vi "Calibration_GUI.vi"() -> ()   [LabVIEW 2012]
uses:
  Custom Controls and Typedefs/Button_GetRefImage.ctl
  Custom Controls and Typedefs/Button_AutoCalibrate.ctl
  Custom Controls and Typedefs/Flip_alongVert_Button.ctl
  Custom Controls and Typedefs/SimulationType.ctl
  Custom Controls and Typedefs/Button_RestoreCalibration.ctl
  Custom Controls and Typedefs/Clear Calibrationctl.ctl
  Custom Controls and Typedefs/CalibrationUI_States.ctl
  Custom Controls and Typedefs/CalibrationType.ctl
  Custom Controls and Typedefs/FGV_CalibrationKeyParams_Actions.ctl
  GFG/GFG Translator Wrapper/GFGTranslator_Action.ctl
  GFG/GFG Translator Wrapper/GFGTranslator_Datatype.ctl
  GFG/GFG Translator Wrapper/GFGTranslator_errors.ctl
  <vilib>/vision/Image Controls.llb/IMAQ Image.ctl
  Custom Controls and Typedefs/Calibration paramaters to Save.ctl
  Custom Controls and Typedefs/Calibration_commonParams.ctl
  SubVIs/Global_CalibrationSimulation.vi
  <vilib>/Utility/config.llb/Read Key (Double).vi
  <vilib>/vision/NI_Vision_Development_Module.lvlib
  GFG/GFG library.lvlib
  <vilib>/Utility/config.llb/NI_LVConfig.lvlib
panel:
  in  "Calibration File I/O":T3
  in  "Auto Refresh?":bool
  in  "Galvo Uncage Path":path=path "D:/Dual Channel Test Images - SciScan/2016_09_20/20160920_11_10_37_galvo_uncage_green_800nm/20160920_11_10_37_galvo_uncage_green_800nm_XYT_ch_1.bmp"
  in  "Reso Image Path":path=path "D:/Dual Channel Test Images - SciScan/2016_09_20/20160920_10_45_54_resonant_800nm_green/20160920_10_45_54_resonant_800nm_green_XYT_ch_1.bmp"
  in  "Galvo Image Path":path=path "D:/Dual Channel Test Images - SciScan/2016_09_20/20160920_11_04_00_galvo_image_green_800nm/20160920_11_04_00_galvo_image_green_800nm_XYT_ch_1.bmp"
  in  "Simulation Type - For Demo ONLY!":T4
  in  "Source Images":T5(tab)
  out "Reference Image (From Uncaging Path)":T6(plugin-control)
  in  "Uncaging Histogram":T7={"auto scale\n      Red "=TRUE, "Min Max (Red)"={0, 2047}, "Histogram"={"Starting Value"=-2011.0, "Incremental Value"=15.722656, "Histogram"=[]}} {"Min Max (Red)" scale=-1921.0..685.0}
  in  "Imaging Path Histogram":T8={"auto scale\n      Blue "=TRUE, "Min Max (Blue)"={0, 2047}, "Histogram"={"Starting Value"=0.0, "Incremental Value"=0.0, "Histogram"=[]}} {"Min Max (Blue)" scale=-32768.0..32767.0}
  out "Imaging Path Image":T6(plugin-control)
  out "Summary":string
  in  "Grab Current Image":T9
  in  "Dial":dbl(knob) scale=-5.0..5.0
  in  "Linear Zoom":cluster{"X.Zoom":dbl, "Y.Zoom":dbl}={"X.Zoom"=1.0, "Y.Zoom"=1.0} {"Y.Zoom" min=1.0 max=5.0 scale=1.0..3.0; "X.Zoom" min=1.0 max=5.0 scale=1.0..3.0}
  in  "Sinusoidal Phase Correction\n(radians)":dbl(slide)=0.6826771653543307 min=0.0 max=1.7 scale=0.0..1.7
  in  "X-Offset (Pixels)":i32(slide) scale=-256.0..256.0
  in  "Y-Offset (Pixels)":i32(slide) scale=256.0..-256.0
  in  "Offset Correction":cluster{"Dummy":dbl}
  in  "Display":enum32{"Image Overlay", "Pixel Mapping"}(tab)
  in  "Blue":bool=TRUE
  in  "Red":bool=TRUE
  out "Red-Blue Overlay":T6(plugin-control)
  out "Relationship between initial pixels and pixels after transformation":cluster{i16[], "Y Indices OUT":i16[]}[](graph)
  in  "reset zoom_Calibration_UI":bool
  in  "Clear All calibrations":bool
  in  "Read Calibration":bool
  out "Y-Pixel Mapping":i16[](array[numeric])
  out "X-Pixel Mapping":i16[](array[numeric])
  in  "Non Linear Stretch":T10={"Phase Offset (2-35%)"=25.0, "Magnitude (0-1)"=0.0} {"Magnitude (0-1)" min=0.0 max=2.0 step=1.0; "Phase Offset (2-35%)" min=2.0 max=50.0}
  in  "Flip":T11
  in  "AutoCalibrate":T12
  # "Red (Stimulation Path)"
  # "Blue (Imaging Path)"
  # "To zoom out press and hold Shift"
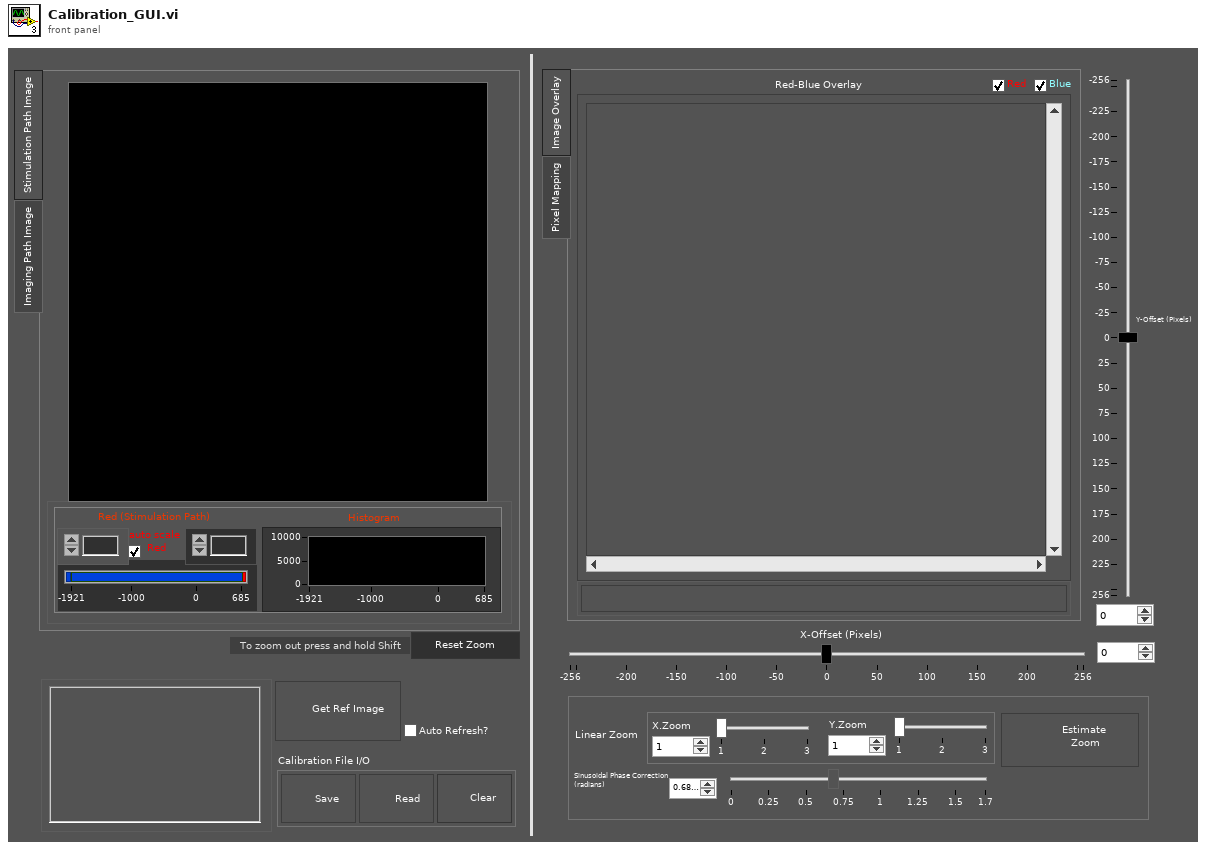
[diagram p1: front panel]
types:
  T1 = typedef "Button_RestoreCalibration.ctl" = bool
  T2 = typedef "Clear Calibrationctl.ctl" = bool
  T3 = cluster{"Save Calibration":bool, "Read Calibration":T1, "Clear Button":T2}
  T4 = typedef "SimulationType.ctl" = enum16{"None", "Uncaging Path Galvo", "Imaging Path Galvo", "Imaging Path Reso"}
  T5 = enum32{"Stimulation Path Image", "Imaging Path Image"}
  T6 = typedef "IMAQ Image.ctl" = refnum<image>
  T7 = cluster{"auto scale\n      Red ":bool, "Min Max (Red)":cluster{i16, i16}, "Histogram":cluster{"Starting Value":sgl, "Incremental Value":sgl, "Histogram":u32[]}}
  T8 = cluster{"auto scale\n      Blue ":bool, "Min Max (Blue)":cluster{i16, i16}, "Histogram":cluster{"Starting Value":sgl, "Incremental Value":sgl, "Histogram":u32[]}}
  T9 = typedef "Button_GetRefImage.ctl" = bool
  T10 = cluster{"Phase Offset (2-35%)":dbl, "Magnitude (0-1)":dbl}
  T11 = typedef "Flip_alongVert_Button.ctl" = bool
  T12 = typedef "Button_AutoCalibrate.ctl" = bool
  T13 = typedef "FGV_CalibrationKeyParams_Actions.ctl" = enum16{"Initialize", "Grab From SciScan and Store", "Read Parameters", "ReadGFGValue"}
  T14 = typedef "CalibrationType.ctl" = enum16{"None", "ImagingGalvoCalibration", "ImagingResoCalibration"}
  T15 = typedef "Image Type" = u32
  T16 = typedef "CalibrationUI_States.ctl" = enum16{"SciScan Disconnected", "Uncaging Galvo", "Imaging Galvo", "Imaging Reso", "Unknown System"}
  T17 = typedef "Calibration paramaters to Save.ctl" = cluster{"General_Parameters":cluster{"SystemType":string, "Date/Time String":string}, "Corection Parameters":cluster{"X-Offset":i32, "Y-Offset":i32, "X-Zoom":dbl, "Y-Zoom":dbl, "PhaseOffset":dbl, "Magnification":dbl, "Flip":bool}, "GFG Params(Numeric)":cluster{"GFG_Varname (Numeric)":string, "GFG_Val (Numeric)":dbl}[]}
  T18 = typedef "GFGTranslator_Datatype.ctl" = enum16{"String", "Path (String)", "Numeric", "Boolean", "Set_BoolRef (use boolean data)", "Get_Variant", "Get_2DArray (I16)", "Get_Image_2DArray (I16)", "Get_Version (String)", "Get_All GFG variables (String)"}
  T19 = typedef "GFGTranslator_Action.ctl" = enum16{"Get", "Set"}
  T20 = typedef "GFGTranslator_errors.ctl" = enum16{"Success", "SciScan Not Running", "No Get Method for Selected Datatype", "No Set Method for Selected Datatype", "Variable Not Found", "Unexpected Datatype", "Data Out of Range"}
  T21 = typedef "Calibration_commonParams.ctl" = cluster{"X.ZOOM.Compensation":dbl, "Y.ZOOM.Compensation":dbl, "Reso_Phase.Correction":dbl}
  T22 = cluster{"Starting Value":sgl, "Incremental Value":sgl, "Histogram":u32[]}
  T23 = typedef "NI_LVConfig.lvlib/Config Data RefNum.ctl" = refnum<k1>
  T24 = cluster{"X-Pixel Mapping":i16[], "Y-Pixel Mapping":i16[]}
  T25 = cluster{"Left (X) pixels dropped":i32, "Right (X) pixels dropped":i32}
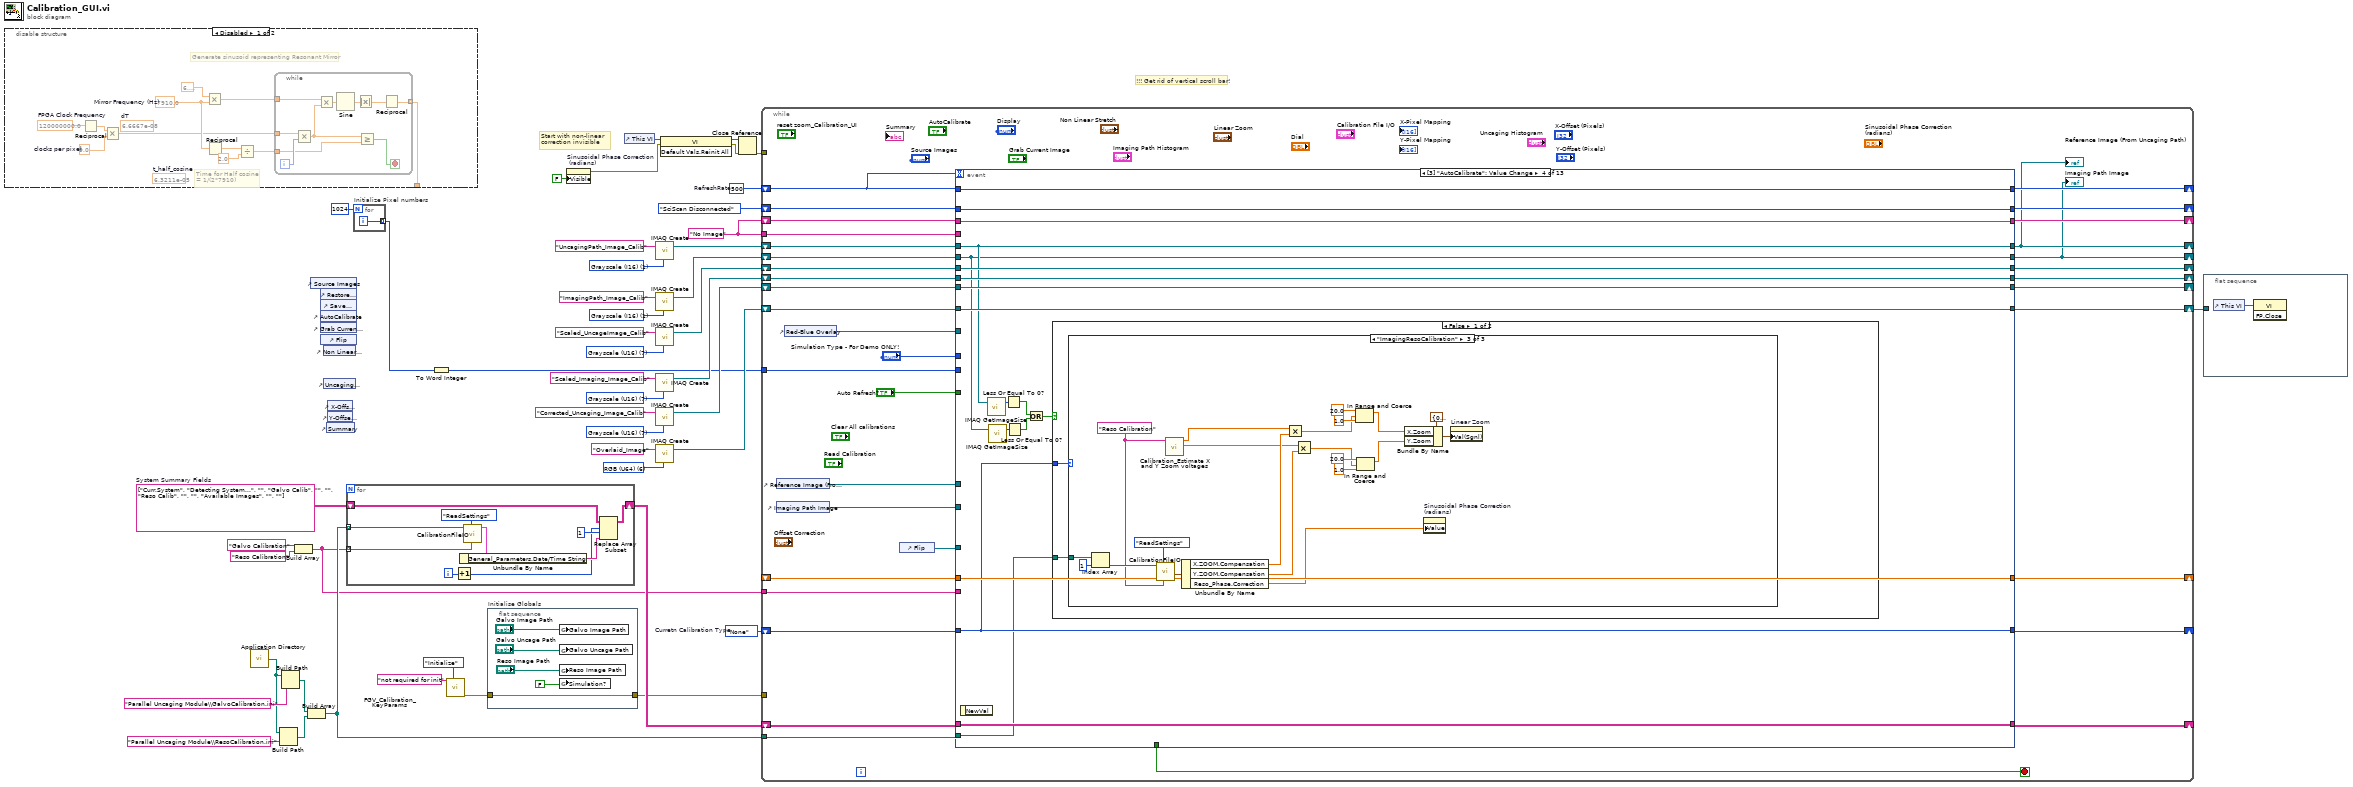
[diagram p0: block diagram]
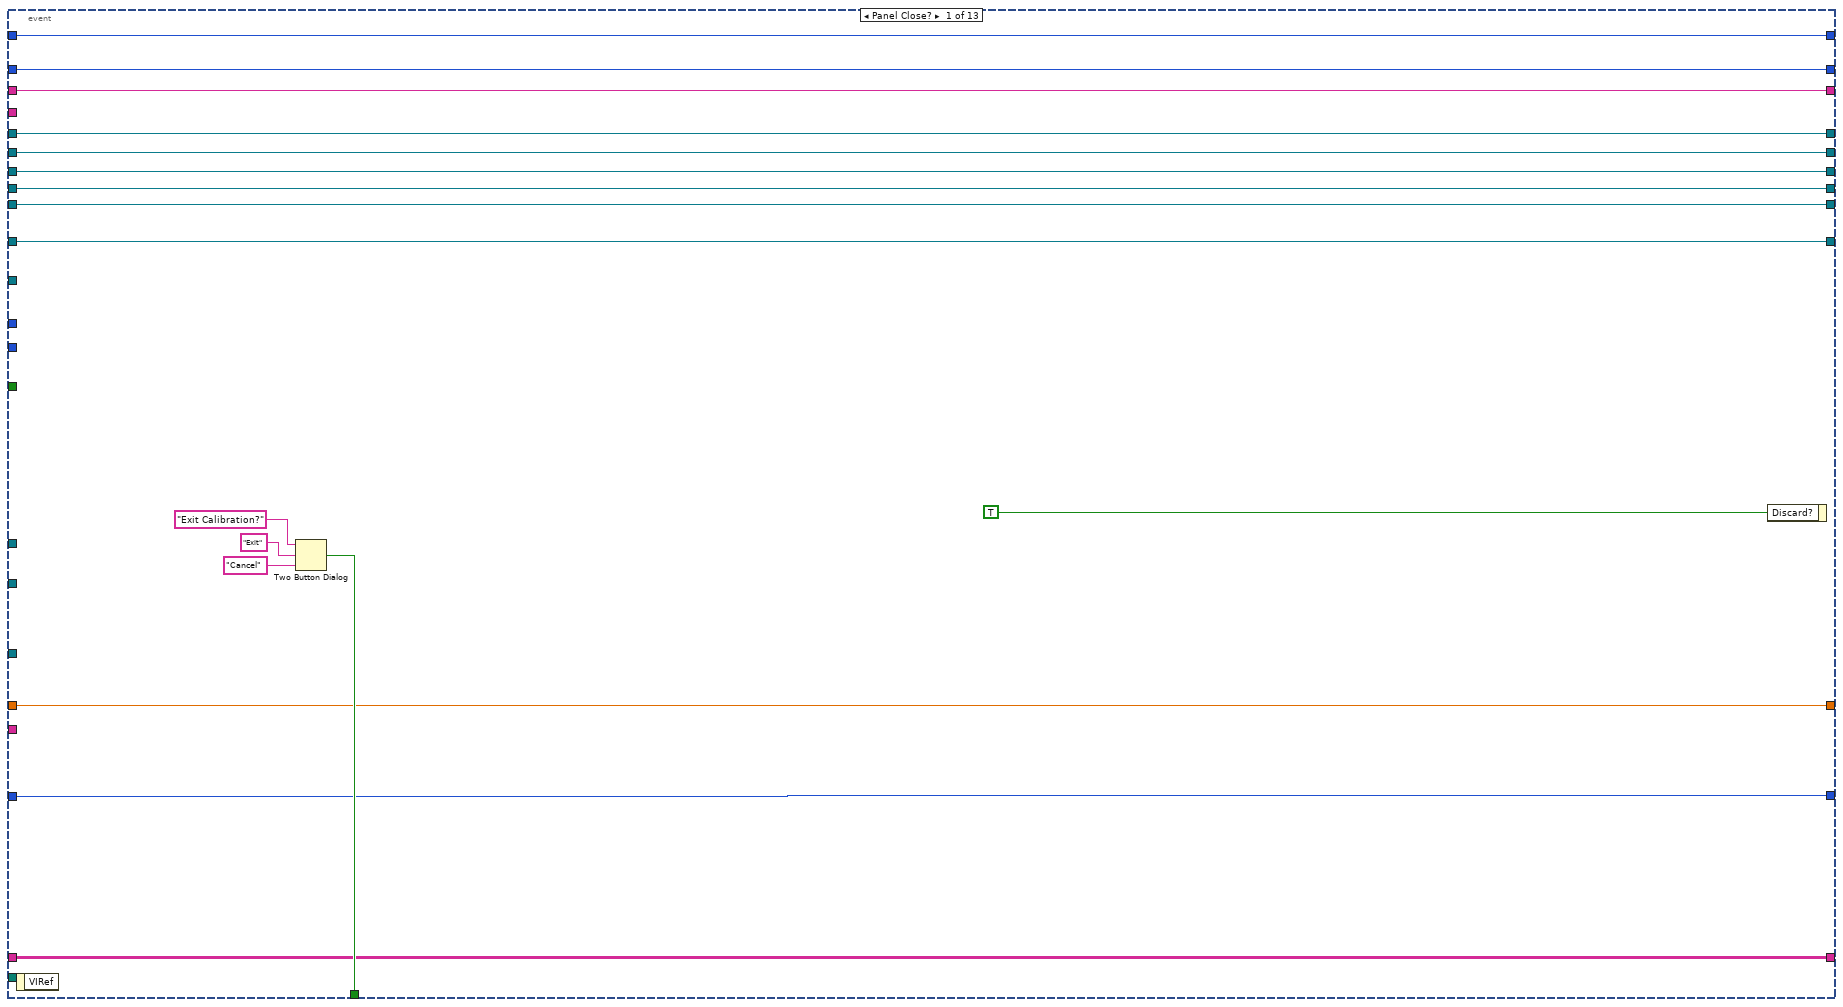
[diagram p3: hidden frame]
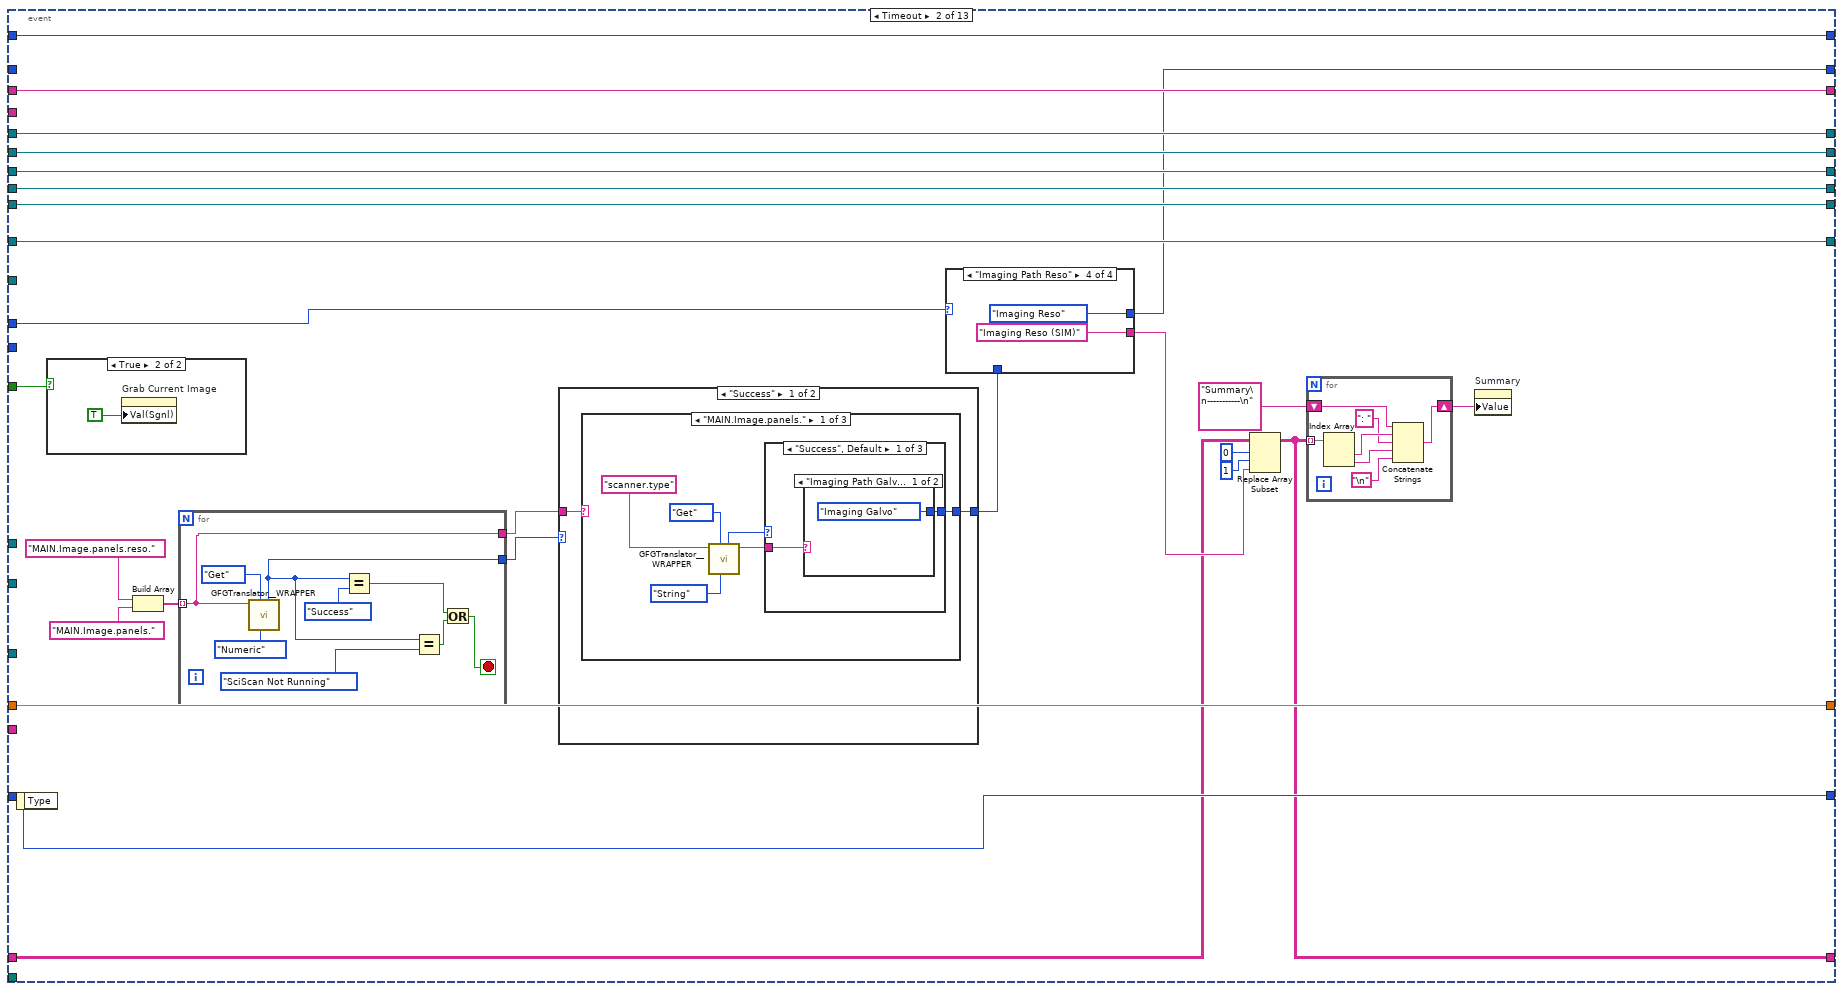
[diagram p4: hidden frame]
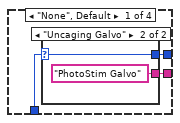
[diagram p5: hidden frame]
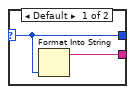
[diagram p6: hidden frame]
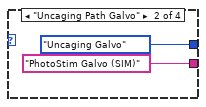
[diagram p7: hidden frame]
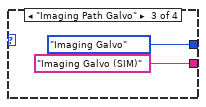
[diagram p8: hidden frame]
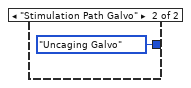
[diagram p10: hidden frame]
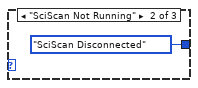
[diagram p11: hidden frame]
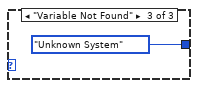
[diagram p12: hidden frame]
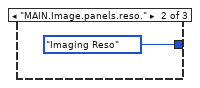
[diagram p13: hidden frame]
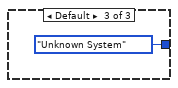
[diagram p14: hidden frame]
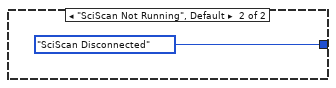
[diagram p15: hidden frame]
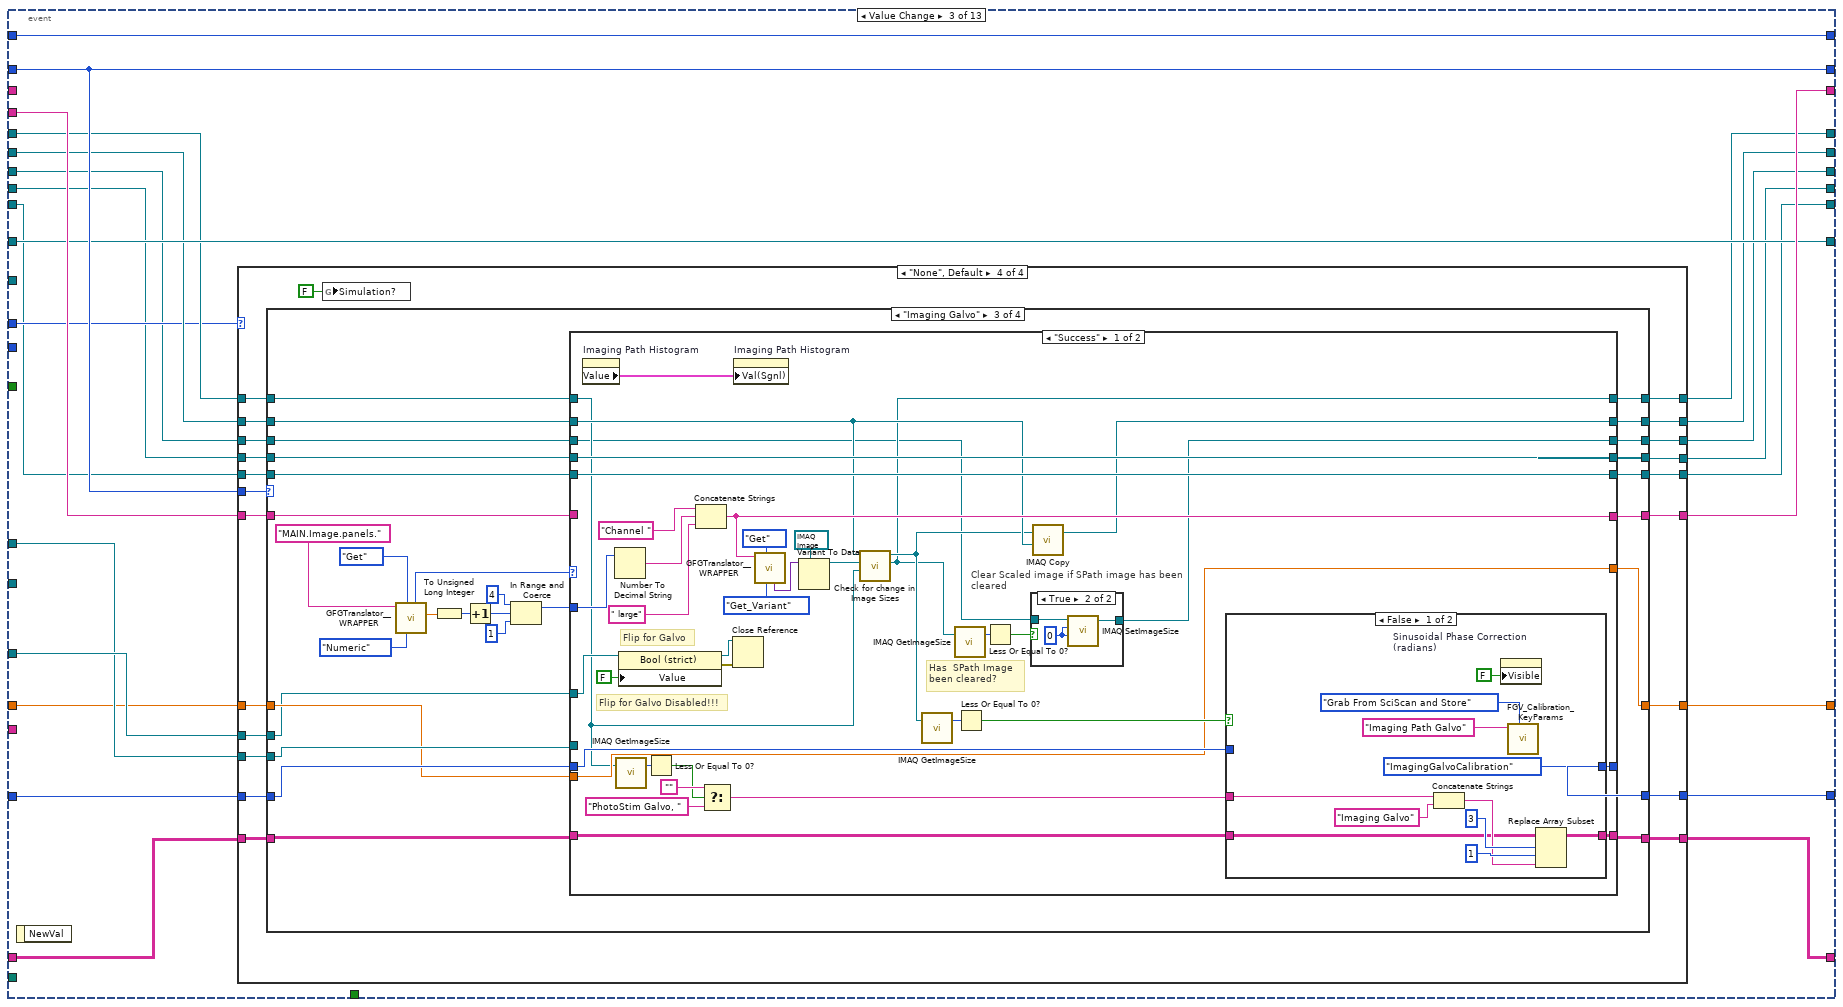
[diagram p16: hidden frame]
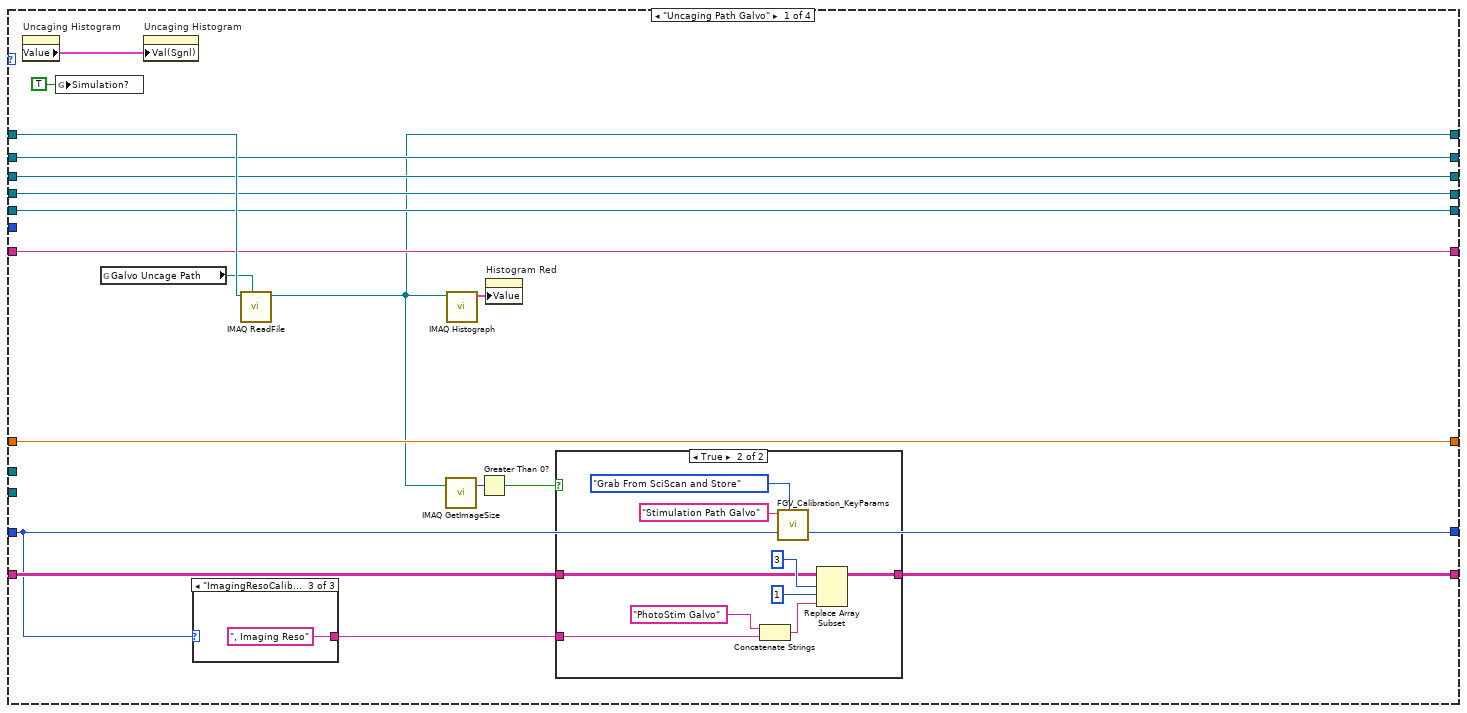
[diagram p17: hidden frame]
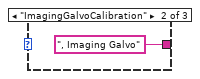
[diagram p20: hidden frame]
diagram:
  w21 = CalibrationType."None"  # Curretn Calibration Type
  w27 = T15 7 items=["Grayscale (U8)", "Grayscale (I16)", "Grayscale (SGL)", "Complex (CSG)", "RGB (U32)", "HSL (U32)", "RGB (U64)", "Grayscale (U16)"] ("Image Type")
  w30 = T15 7 items=["Grayscale (U8)", "Grayscale (I16)", "Grayscale (SGL)", "Complex (CSG)", "RGB (U32)", "HSL (U32)", "RGB (U64)", "Grayscale (U16)"] ("Image Type")
  w32 = T15 7 items=["Grayscale (U8)", "Grayscale (I16)", "Grayscale (SGL)", "Complex (CSG)", "RGB (U32)", "HSL (U32)", "RGB (U64)", "Grayscale (U16)"] ("Image Type")
  w36 = T15 1 items=["Grayscale (U8)", "Grayscale (I16)", "Grayscale (SGL)", "Complex (CSG)", "RGB (U32)", "HSL (U32)", "RGB (U64)", "Grayscale (U16)"] ("Image Type")
  w38 = T15 6 items=["Grayscale (U8)", "Grayscale (I16)", "Grayscale (SGL)", "Complex (CSG)", "RGB (U32)", "HSL (U32)", "RGB (U64)", "Grayscale (U16)"] ("Image Type")
  w39 = T15 1 items=["Grayscale (U8)", "Grayscale (I16)", "Grayscale (SGL)", "Complex (CSG)", "RGB (U32)", "HSL (U32)", "RGB (U64)", "Grayscale (U16)"] ("Image Type")
  w42 = "No Image"
  w44 = string[][] [["Curr.System", "Detecting System...", ""], ["Galvo Calib", "", ""], ["Reso Calib", "", ""], ["Available Images", "", ""]]  # System Summary Fields
  w47 = 500  # RefreshRate
  # "Start with non-linear correction invisible"
  # "!!! Get rid of vertical scroll bar!"
  n1 = disable-structure shown="Disabled" {
    disable-tunnel: [w48 _] -> _
    frame Disabled {
      w50 = 9.0  # clocks per pixel
      w52 = 120000000.0  # FPGA Clock Frequency
      w54 = 7910.0  # Mirror Frequency (Hz)
      (unwired) 6.6667e-08  # dT
      (unwired) 6.3211e-05  # t_half_cosine
      # "Generate sinusoid representing Resonant Mirror"
      # "Time for Half cosine\n= 1/(2*7910)"
      n2 = Reciprocal(x=w52) -> (1/x=w51:dbl)
      n3 = Multiply(x=w51, y=w50) -> (x*y=w49:dbl)
      n4 = Multiply(x=6.283185307179586, y=w54) -> (x*y=w57:dbl)
      n5 = Reciprocal(x=w54) -> (1/x=w55:dbl)
      n6 = Divide(x=w55, y=2.0) -> (x/y=w53:dbl)
      n7 = while {
        tunnel: w49 -> [w67]
        tunnel: w57 -> [w64]
        tunnel: w53 -> [w66]
        tunnel: [w60] -> w48 mode=indexing
        i -> [w68]
        stop <- w65 stop-if-true
        n8 = Multiply(x=w67, y=w68) -> (x*y=w63:dbl)
        n9 = Multiply(x=w64, y=w63) -> (x*y=w62:dbl)
        n10 = Sine(x=w62) -> (sin(x)=w61:dbl)
        n11 = Absolute Value(x=w61) -> (abs(x)=w59:dbl)
        n12 = Greater Or Equal?(x=w63, y=w66) -> (x >= y?=w65:bool)
        n13 = Reciprocal(x=w59) -> (1/x=w60:dbl)
      }
    }
    frame Enabled {
    }
  }
  n14 = call <vilib>:"Application Directory.vi"() -> ("Application Directory"=w23:path)
  n15 = Build Path(base path=w23, name or relative path="Parallel Uncaging Module\\ResoCalibration.ini") -> (appended path=w19:path)
  n16 = Build Path(base path=w23, name or relative path="Parallel Uncaging Module\\GalvoCalibration.ini") -> (appended path=w20:path)
  n17 = Build Array("Galvo Calibration" ("Calibration Type"), "Reso Calibration" ("Calibration Type")) -> (w6:string[])
  n18 = Build Array(w20, w19) -> (w45:path[])
  n19 = control-ref of="Source Images"() -> ()  [unwired: 1 out]
  n20 = control-ref of="Restore Calibration"() -> ()  [unwired: 1 out]
  n21 = control-ref of="Save Calibration"() -> ()  [unwired: 1 out]
  n22 = control-ref of="AutoCalibrate"() -> ()  [unwired: 1 out]
  n23 = control-ref of="Grab Current Image"() -> ()  [unwired: 1 out]
  n24 = control-ref of="Flip"() -> ()  [unwired: 1 out]
  n25 = control-ref of="Non Linear Stretch"() -> ()  [unwired: 1 out]
  n26 = control-ref of="Uncaging Histogram"() -> ()  [unwired: 1 out]
  n27 = control-ref of="Summary"() -> ()  [unwired: 1 out]
  n28 = control-ref of="X-Offset (Pixels)"() -> ()  [unwired: 1 out]
  n29 = control-ref of="Y-Offset (Pixels)"() -> ()  [unwired: 1 out]
  n30 = for {
    tunnel: w45 -> [w70] mode=indexing
    shift-right: [w72] -> w43
    shift-left: w44 -> [w76]
    tunnel: w6 -> [w69] mode=indexing
    i -> [w75]
    n31 = Increment(x=w75) -> (x+1=w71:i32)
    n32 = call "CalibrationFileIO.vi"("Calibration Type"=w69, "CalibrationFileIO_command"=enum16{"WriteSettings", "ReadSettings"}."ReadSettings", "configuration file path"=w70) -> ("Calibration paramaters_OUT"=w77:T17)  [unwired: 6 in, 2 out]
    n33 = Unbundle By Name(w77) -> ("General_Parameters.Date/Time String"=w73:string)
    n34 = Replace Array Subset(array=w76, new element=w73, index (row)=w71, index (col)=1 ("disabled index (col)")) -> (w72:string[][])
  }
  n35 = for "Initialize Pixel numbers" {
    N: 1024 -> [_]
    tunnel: [w79] -> w2 mode=indexing
    i -> [w79]
  }
  n36 = To Word Integer(number=w2) -> (16bit integer=w1:i16[])
  n37 = call "FGV_Calibration_KeyParams.vi"("Action"=FGV_CalibrationKeyParams_Actions."Initialize", "System Type"="not required for init") -> ("error out"=w12:errorcluster)  [unwired: 4 in, 5 out]
  n38 = flat-sequence "Initialise Globals" {
    tunnel: w12 -> [w80]
    tunnel: [w80] -> w11
    frame #0 {
      n39 = global write "Global_CalibrationSimulation.vi" "Galvo Image Path"("Galvo Image Path") -> ()
      n40 = global write "Global_CalibrationSimulation.vi" "Galvo Uncage Path"("Galvo Uncage Path") -> ()
      n41 = global write "Global_CalibrationSimulation.vi" "Reso Image Path"("Reso Image Path") -> ()
      n42 = global write "Global_CalibrationSimulation.vi" "Simulation?"(FALSE) -> ()
    }
  }
  n43 = property on="Sinusoidal Phase Correction\n (radians)" class="Slide (strict)"("Visible"=FALSE) -> (error out=w3:errorcluster)  [unwired: 2 in, 1 out]
  n44 = control-ref of="This VI"() -> (w16:refnum<vi>)
  n45 = call "IMAQ Create"("Image Name"="UncagingPath_Image_Calib", "Image Type"=w39) -> ("New Image"=w37:T6)  [unwired: 3 in, 1 out]
  n46 = call "IMAQ Create"("Image Name"="ImagingPath_Image_Calib", "Image Type"=w36) -> ("New Image"=w17:T6)  [unwired: 3 in, 1 out]
  n47 = call "IMAQ Create"("Image Name"="Scaled_UncageImage_Calib", "Image Type"=w32) -> ("New Image"=w31:T6)  [unwired: 3 in, 1 out]
  n48 = call "IMAQ Create"("Image Name"="Scaled_Imaging_Image_Calib", "Image Type"=w30) -> ("New Image"=w28:T6)  [unwired: 3 in, 1 out]
  n49 = call "IMAQ Create"("Image Name"="Corrected_Uncaging_Image_Calib", "Image Type"=w27) -> ("New Image"=w25:T6)  [unwired: 3 in, 1 out]
  n50 = call "IMAQ Create"("Image Name"="Overlaid_Image", "Image Type"=w38) -> ("New Image"=w34:T6)  [unwired: 3 in, 1 out]
  n51 = invoke class="VI" method="Default Vals.Reinit All"(reference=w16, error in=w3) -> (reference out=w15:refnum<vi>, error out=w14:errorcluster)  [unwired: 1 in, 1 out]
  n52 = Close Reference(reference=w15, error in (no error)=w14) -> (error out=w13:errorcluster)
  n53 = while {
    shift-right: [w118] -> _
    shift-left: w47 -> [w117]
    shift-right: [w114] -> _
    shift-left: CalibrationUI_States."SciScan Disconnected" -> [w116]
    tunnel: w45 -> [w115]
    shift-right: [w112] -> _
    shift-left: w43 -> [w113]
    shift-right: [w111] -> _
    shift-left: w42 -> [w110]
    tunnel: w42 -> [w109]
    shift-right: [w91] -> w18
    shift-left: w34 -> [w106]
    shift-right: [w89] -> _
    shift-left: w17 -> [w107]
    shift-right: [w90] -> _
    shift-left: w37 -> [w108]
    shift-right: [w100] -> _
    shift-left: w31 -> [w105]
    shift-right: [w101] -> _
    shift-left: w28 -> [w103]
    shift-right: [w99] -> _
    shift-left: w25 -> [w102]
    shift-right: [w96] -> _
    shift-left: w21 -> [w97]
    shift-right: [w93] -> _
    shift-left: _ -> [w92]
    tunnel: w13 -> [_]
    tunnel: w11 -> [_]
    tunnel: w6 -> [w88]
    tunnel: w1 -> [w86]
    stop <- w119 stop-if-true
    n54 = control-ref of="Reference Image (From Uncaging Path)"() -> (w94:refnum<vi>)
    n55 = control-ref of="Imaging Path Image"() -> (w87:refnum<vi>)
    n56 = control-ref of="Red-Blue Overlay"() -> (w85:refnum<vi>)
    n57 = control-ref of="Flip"() -> (w98:refnum<vi>)
    n58 = event shown="[3] \"AutoCalibrate\": Value Change" {
      selector: _ -> [_ _ _ _ _ _ _ _ _ _ _ _ _]
      dyn-events: _ -> [_ _ _ _ _ _ _ _ _ _ _ _ _]
      timeout: w117 -> [_ _ _ _ _ _ _ _ _ _ _ _ _]
      tunnel: [w133 _ _ _ _ _ _ _ _ _ _ _ _] -> w119
      tunnel: [w132 w162 w233 w695 w756 w785 w900 w929 w952 w1095 w1162 w1265 w1281] -> w118
      tunnel: w117 -> [w132 w162 w233 w695 w756 w785 w900 w929 w952 w1095 w1162 w1265 w1281]
      tunnel: w116 -> [w130 _ w232 w694 w755 w784 w899 w928 w951 w1094 w1146 w1264 w1280]
      tunnel: w115 -> [_ _ _ w678 _ w777 w891 _ _ _ _ _ w1269]
      tunnel: [w130 w142 w232 w694 w755 w784 w899 w928 w951 w1094 w1146 w1264 w1280] -> w114
      tunnel: w113 -> [w129 w137 w214 w693 w754 w775 w898 w927 w950 w1093 w1161 w1263 w1267]
      tunnel: [w129 w139 w213 w693 w754 w774 w898 w927 w950 w1093 w1161 w1263 w1266] -> w112
      tunnel: [w128 w154 w231 w692 w753 w783 w897 w926 w949 w1092 w1160 w1262 w1279] -> w111
      tunnel: w110 -> [w128 w154 _ w692 w753 w783 w897 w926 w949 w1092 w1160 w1262 w1279]
      tunnel: w109 -> [_ _ w230 _ _ _ _ _ _ _ _ _ _]
      tunnel: w108 -> [w127 w153 w228 w685 w752 w782 w884 w925 w946 w1089 w1159 w1261 w1278]
      tunnel: w107 -> [w126 w152 w227 w683 w751 w781 w885 w924 w948 w1067 w1158 w1260 w1277]
      tunnel: w106 -> [w125 w151 w229 w691 w750 w780 w896 w923 w942 w1091 w1151 w1259 w1276]
      tunnel: [w127 w153 w225 w685 w752 w782 w884 w925 w946 w1089 w1159 w1261 w1278] -> w90
      tunnel: [w126 w152 w226 w683 w751 w781 w885 w924 w948 w1068 w1158 w1260 w1277] -> w89
      tunnel: [w125 w151 w229 w691 w750 w780 w896 w923 w942 w1091 w1144 w1259 w1276] -> w91
      tunnel: w105 -> [w124 w150 w222 w690 w749 w772 w895 w922 w941 w1085 w1156 w1258 w1275]
      tunnel: [w124 w150 w221 w690 w749 w772 w895 w922 w939 w1085 w1156 w1258 w1275] -> w100
      tunnel: "Simulation Type - For Demo ONLY!" -> [_ w144 w224 _ _ _ _ _ _ _ _ _ _]
      tunnel: w103 -> [w123 w149 w223 w689 w748 w771 w894 w921 w943 w1077 w1149 w1257 w1274]
      tunnel: [w123 w149 w220 w689 w748 w771 w894 w921 w943 w1084 w1149 w1257 w1274] -> w101
      tunnel: w102 -> [w122 w148 w219 w688 w747 w779 w893 w920 w940 w1083 w1154 w1256 w1273]
      tunnel: [w122 w148 w218 w688 w747 w779 w893 w920 w938 w1083 w1150 w1256 w1273] -> w99
      tunnel: w98 -> [_ _ w217 _ _ w776 _ _ w934 w1079 _ w1252 _]
      tunnel: w97 -> [w121 w147 w215 w679 w746 w778 w875 w919 w933 w1063 w1145 w1251 w1272]
      tunnel: [w121 w147 w216 w679 w746 w778 w875 w919 w933 w1063 w1145 w1251 w1272] -> w96
      tunnel: "Auto Refresh?" -> [_ w146 _ _ _ _ _ _ _ _ _ _ _]
      tunnel: w94 -> [_ _ w212 _ w742 _ _ _ w931 _ _ _ _]
      tunnel: [w120 w145 w211 w687 w745 w773 w888 w918 w932 w1078 w1143 w1250 w1271] -> w93
      tunnel: w92 -> [w120 w145 w210 w687 w745 w773 w888 w918 w932 w1078 w1143 w1250 w1271]
      tunnel: w88 -> [_ _ _ _ _ w761 w887 _ _ _ _ _ _]
      tunnel: w87 -> [_ _ _ _ w743 _ _ _ _ _ _ _ _]
      tunnel: w86 -> [_ _ _ _ _ _ _ _ _ _ w1142 _ _]
      tunnel: w85 -> [_ _ _ _ w740 _ _ _ _ _ _ _ _]
      event Panel Close? {
        n59 = event-data() -> ()  [unwired: 1 in, 1 out]
        n60 = Two Button Dialog(message="Exit Calibration?", 1:"Cancel" ("F button name (\"Cancel\")"), 2:"Exit" ("T button name (\"OK\")")) -> (T button?=w133:bool)
        n61 = event-data("Discard?"=TRUE) -> ()  [unwired: 1 in, 1 out]
      }
      event Timeout {
        n62 = event-data() -> ()  [unwired: 1 in, 1 out]
        n63 = case shown="True" w146 {
          frame False {
          }
          frame True {
            n64 = property on="Grab Current Image" class="Bool"("Val(Sgnl)"=TRUE) -> ()  [unwired: 2 in, 2 out]
          }
        }
        n65 = Build Array("MAIN.Image.panels.reso." ("GFG Variable Name"), "MAIN.Image.panels." ("GFG Variable Name")) -> (w159:string[])
        n66 = for {
          tunnel: [w206] -> w158
          tunnel: w159 -> [w201] mode=indexing
          tunnel: [w201] -> w157
          stop <- w202 stop-if-true
          n67 = call "GFGTranslator__WRAPPER.vi"("GFGTranslator Datatype"=GFGTranslator_Datatype."Numeric", "GFG Translator Action"=GFGTranslator_Action."Get", "GFG Variable Name"=w201) -> ("Status Output"=w206:T20)  [unwired: 3 in, 5 out]
          n68 = Equal?(x=w206, y=GFGTranslator_errors."Success") -> (x = y?=w203:bool)
          n69 = Equal?(x=w206, y=GFGTranslator_errors."SciScan Not Running") -> (x = y?=w204:bool)
          n70 = Or(x=w203, y=w204) -> (x .or. y?=w202:bool)
        }
        n71 = case shown="\"Success\"" w158 {
          tunnel: [w184 CalibrationUI_States."SciScan Disconnected"] -> w143
          tunnel: w157 -> [w185 _]
          frame "Success" {
            n72 = case shown="\"MAIN.Image.panels.\"" w185 {
              tunnel: [w187 CalibrationUI_States."Imaging Reso" CalibrationUI_States."Unknown System"] -> w184
              frame "MAIN.Image.panels." {
                n73 = call "GFGTranslator__WRAPPER.vi"("GFGTranslator Datatype"=GFGTranslator_Datatype."String", "GFG Translator Action"=GFGTranslator_Action."Get", "GFG Variable Name"="scanner.type") -> ("String_Output"=w186:string, "Status Output"=w188:T20)  [unwired: 3 in, 4 out]
                n74 = case shown="\"Success\", Default" w188 {
                  tunnel: [w193 CalibrationUI_States."SciScan Disconnected" CalibrationUI_States."Unknown System"] -> w187
                  tunnel: w186 -> [w192 _ _]
                  frame "Success", Default {
                    n75 = case shown="\"Imaging Path Galvo\", Default" w192 {
                      tunnel: [CalibrationUI_States."Imaging Galvo" CalibrationUI_States."Uncaging Galvo"] -> w193
                      frame "Imaging Path Galvo", Default {
                      }
                      frame "Stimulation Path Galvo" {
                      }
                    }
                  }
                  frame "SciScan Not Running" {
                  }
                  frame "Variable Not Found" {
                  }
                }
              }
              frame "MAIN.Image.panels.reso." {
              }
              frame Default {
              }
            }
          }
          frame "SciScan Not Running", Default {
          }
        }
        n76 = case shown="\"Imaging Path Reso\"" w144 {
          tunnel: [w163 CalibrationUI_States."Uncaging Galvo" CalibrationUI_States."Imaging Galvo" CalibrationUI_States."Imaging Reso"] -> w142
          tunnel: w143 -> [w165 _ _ _]
          tunnel: [w164 "PhotoStim Galvo (SIM)" ("GFG Variable Name") "Imaging Galvo (SIM)" ("GFG Variable Name") "Imaging Reso (SIM)" ("GFG Variable Name")] -> w138
          frame "None", Default {
            n77 = case shown="\"Uncaging Galvo\"" w165 {
              selector: w165 -> [w167 w168]
              tunnel: [w166 "PhotoStim Galvo" ("GFG Variable Name")] -> w164
              tunnel: [w167 w168] -> w163
              frame Default {
                n78 = Format Into String(w167) -> (resulting string=w166:string)  [unwired: 3 in, 1 out]
              }
              frame "Uncaging Galvo" {
              }
            }
          }
          frame "Uncaging Path Galvo" {
          }
          frame "Imaging Path Galvo" {
          }
          frame "Imaging Path Reso" {
          }
        }
        n79 = Replace Array Subset(array=w137, new element=w138, index (row)=0, index (col)=1 ("disabled index (col)")) -> (w139:string[][])
        n80 = for {
          tunnel: w139 -> [w183] mode=indexing
          shift-right: [w177] -> w156
          shift-left: "Summary\n-----------\n" ("GFG Variable Name") -> [w178]
          n81 = Index Array(array=w183) -> (element #1=w182:string, element #2=w180:string)  [unwired: 2 in]
          n82 = Concatenate Strings(w178, w182, ": " ("string"), w180, "\n") -> (w177:string)
        }
        n83 = property on="Summary" class="Str"("Value"=w156) -> ()  [unwired: 2 in, 2 out]
      }
      event Value Change {
        n84 = event-data() -> ()  [unwired: 1 in, 1 out]
        n85 = case shown="\"None\", Default" w224 {
          tunnel: w232 -> [_ _ _ w381]
          tunnel: [w249 w285 w326 w380] -> w231
          tunnel: w230 -> [w249 w285 w326 w379]
          tunnel: w228 -> [w251 w268 w308 w378]
          tunnel: w227 -> [w250 w284 w325 w377]
          tunnel: [w250 w271 w311 w376] -> w226
          tunnel: [w236 w268 w308 w375] -> w225
          tunnel: w222 -> [w247 w282 w323 w374]
          tunnel: w223 -> [w246 w283 w324 w371]
          tunnel: [w247 w282 w323 w373] -> w221
          tunnel: [w246 w283 w324 w372] -> w220
          tunnel: w219 -> [w245 w280 w321 w369]
          tunnel: [w245 w280 w321 w370] -> w218
          tunnel: w217 -> [_ w273 w313 w368]
          tunnel: [w243 w279 w320 w367] -> w216
          tunnel: w215 -> [w243 w269 w309 w366]
          tunnel: w214 -> [w244 w278 w319 w365]
          tunnel: [w241 w277 w318 w364] -> w213
          tunnel: w212 -> [_ _ _ w363]
          tunnel: [w240 w264 w305 w362] -> w211
          tunnel: w210 -> [w240 w264 w304 w361]
          frame "Uncaging Path Galvo" {
            n86 = property on="Uncaging Histogram" class="Clust (strict)"() -> ("Value"=w239:T7)  [unwired: 2 in, 2 out]
            n87 = global write "Global_CalibrationSimulation.vi" "Simulation?"(TRUE ("Simulation?")) -> ()
            n88 = global read "Global_CalibrationSimulation.vi" "Galvo Uncage Path"() -> (w237:path)
            n89 = property on="Uncaging Histogram" class="Clust (strict)"("Val(Sgnl)"=w239) -> ()  [unwired: 2 in, 2 out]
            n90 = case shown="\"ImagingResoCalibration\"" w243 {
              tunnel: [_ ", Imaging Galvo" ("regular expression") ", Imaging Reso" ("regular expression")] -> w242
              frame "None", Default {
              }
              frame "ImagingGalvoCalibration" {
              }
              frame "ImagingResoCalibration" {
              }
            }
            n91 = call "IMAQ ReadFile"("File Path"=w237, "Image"=w251) -> ("Image Out"=w236:T6)  [unwired: 5 in, 4 out]
            n92 = call "IMAQ GetImageSize"("Image"=w236) -> ("Y Resolution"=w235:i32)  [unwired: 3 in, 2 out]
            n93 = call "IMAQ Histograph"("Image"=w236) -> ("Histogram Graph"=w248:T22)  [unwired: 7 in, 3 out]
            n94 = Greater Than 0?(x=w235) -> (x > 0?=w234:bool)
            n95 = property on="Histogram Red" class="WFGraph (strict)"("Value"=w248) -> ()  [unwired: 2 in, 2 out]
            n96 = case shown="True" w234 {
              tunnel: w244 -> [w252 w259]
              tunnel: w242 -> [_ w257]
              tunnel: [w252 w255] -> w241
              frame False {
              }
              frame True {
                n97 = Concatenate Strings("PhotoStim Galvo" ("regular expression"), w257) -> (w256:string)
                n98 = call "FGV_Calibration_KeyParams.vi"("Action"=FGV_CalibrationKeyParams_Actions."Grab From SciScan and Store", "System Type"="Stimulation Path Galvo") -> ()  [unwired: 4 in, 6 out]
                n99 = Replace Array Subset(array=w259, new element=w256, index (row)=3, index (col)=1 ("disabled index (col)")) -> (w255:string[][])
              }
            }
          }
          frame "Imaging Path Galvo" {
            # "Apply Flip for Galvo"
            n100 = property on="Imaging Path Histogram" class="Clust (strict)"() -> ("Value"=w266:T8)  [unwired: 2 in, 2 out]
            n101 = global read "Global_CalibrationSimulation.vi" "Galvo Image Path"() -> (w265:path)
            n102 = global write "Global_CalibrationSimulation.vi" "Simulation?"(TRUE ("Simulation?")) -> ()
            n103 = property class="Bool (strict)"(reference=w273, "Value"=T11 TRUE) -> (reference out=w274:refnum<vi>, error out=w275:errorcluster)  [unwired: 1 in]
            n104 = property on="Imaging Path Histogram" class="Clust (strict)"("Val(Sgnl)"=w266) -> ()  [unwired: 2 in, 2 out]
            n105 = call "IMAQ ReadFile"("File Path"=w265, "Image"=w284) -> ("Image Out"=w271:T6)  [unwired: 5 in, 4 out]
            n106 = Close Reference(reference=w274, error in (no error)=w275) -> ()  [unwired: 1 out]
            n107 = call "IMAQ GetImageSize"("Image"=w271) -> ("X Resolution"=w272:i32)  [unwired: 3 in, 2 out]
            n108 = Greater Than 0?(x=w272) -> (x > 0?=w270:bool)
            n109 = call "IMAQ Histograph"("Image"=w271) -> ("Histogram Graph"=w281:T22)  [unwired: 7 in, 3 out]
            n110 = property on="Histogram" class="WFGraph (strict)"("Value"=w281) -> ()  [unwired: 2 in, 2 out]
            n111 = case shown="True" w270 {
              tunnel: [w287 w303] -> w279
              tunnel: w278 -> [w286 w298]
              tunnel: [w286 w297] -> w277
              tunnel: w269 -> [w287 _]
              tunnel: w268 -> [_ w291]
              frame False {
              }
              frame True {
                w303 = CalibrationType."ImagingGalvoCalibration"  # Curretn Calibration Type
                n112 = property on="Sinusoidal Phase Correction\n(radians)" class="Slide (strict)"("Visible"=FALSE) -> ()  [unwired: 2 in, 2 out]
                n113 = call "IMAQ GetImageSize"("Image"=w291) -> ("X Resolution"=w293:i32)  [unwired: 3 in, 2 out]
                n114 = Greater Than 0?(x=w293) -> (x > 0?=w294:bool)
                n115 = Select(t="PhotoStim Galvo, " ("regular expression"), s=w294, f="") -> (s? t:f=w292:string)
                n116 = Concatenate Strings(w292, "Imaging Galvo" ("regular expression")) -> (w300:string)
                n117 = call "FGV_Calibration_KeyParams.vi"("Action"=FGV_CalibrationKeyParams_Actions."Grab From SciScan and Store", "System Type"="Imaging Path Galvo") -> ()  [unwired: 4 in, 6 out]
                n118 = Replace Array Subset(array=w298, new element=w300, index (row)=3, index (col)=1 ("disabled index (col)")) -> (w297:string[][])
              }
            }
          }
          frame "Imaging Path Reso" {
            # "No flip for Reso"
            n119 = global read "Global_CalibrationSimulation.vi" "Reso Image Path"() -> (w306:path)
            n120 = global write "Global_CalibrationSimulation.vi" "Simulation?"(TRUE ("Simulation?")) -> ()
            n121 = property on="Imaging Path Histogram" class="Clust (strict)"() -> ("Value"=w317:T8)  [unwired: 2 in, 2 out]
            n122 = property class="Bool (strict)"(reference=w313, "Value"=T11 FALSE) -> (reference out=w314:refnum<vi>, error out=w315:errorcluster)  [unwired: 1 in]
            n123 = call "IMAQ ReadFile"("File Path"=w306, "Image"=w325) -> ("Image Out"=w311:T6)  [unwired: 5 in, 4 out]
            n124 = Close Reference(reference=w314, error in (no error)=w315) -> ()  [unwired: 1 out]
            n125 = property on="Imaging Path Histogram" class="Clust (strict)"("Val(Sgnl)"=w317) -> ()  [unwired: 2 in, 2 out]
            n126 = call "IMAQ GetImageSize"("Image"=w311) -> ("X Resolution"=w312:i32)  [unwired: 3 in, 2 out]
            n127 = Greater Than 0?(x=w312) -> (x > 0?=w310:bool)
            n128 = case shown="True" w310 {
              tunnel: [w329 CalibrationType."ImagingResoCalibration" ("Curretn Calibration Type")] -> w320
              tunnel: w319 -> [w328 w355]
              tunnel: [w328 w354] -> w318
              tunnel: w309 -> [w329 _]
              tunnel: w308 -> [_ w347]
              tunnel: w306 -> [_ w333]
              tunnel: [w327 w332] -> w305
              tunnel: w304 -> [w327 _]
              frame False {
              }
              frame True {
                n129 = call "IMAQ GetImageSize"("Image"=w347) -> ("X Resolution"=w349:i32)  [unwired: 3 in, 2 out]
                n130 = Greater Than 0?(x=w349) -> (x > 0?=w350:bool)
                n131 = Strip Path(path=w333) -> (stripped path=w340:path, name=w342:string)
                n132 = Select(t="PhotoStim Galvo, " ("regular expression"), s=w350, f="") -> (s? t:f=w348:string)
                n133 = Match Pattern(string=w342, regular expression="_ch" ("search string")) -> (before substring=w341:string)  [unwired: 1 in, 3 out]
                n134 = Concatenate Strings(w341, ".INI" ("string")) -> (w339:string)
                n135 = Build Path(base path=w340, name or relative path=w339) -> (appended path=w338:path)
                n136 = call <vilib>:"Open Config Data.vi"("configuration file path"=w338) -> ("refnum"=w337:T23)  [unwired: 8 in, 2 out]
                n137 = Concatenate Strings(w348, "Imaging Reso" ("regular expression")) -> (w357:string)
                n138 = call "FGV_Calibration_KeyParams.vi"("Action"=FGV_CalibrationKeyParams_Actions."Grab From SciScan and Store", "System Type"="Imaging Path Reso") -> ()  [unwired: 4 in, 6 out]
                n139 = call-poly <vilib>:"Read Key.vi"("section"="_", "key"="Start.Delay", "refnum"=w337) -> ("error out"=w335:errorcluster, "value"=w332:dbl, "refnum out"=w334:T23)  [unwired: 5 in, 1 out]
                n140 = Replace Array Subset(array=w355, new element=w357, index (row)=3, index (col)=1 ("disabled index (col)")) -> (w354:string[][])
                n141 = call <vilib>:"Close Config Data.vi"("error in (no error)"=w335, "refnum"=w334) -> ()  [unwired: 8 in, 2 out]
                n142 = property on="Sinusoidal Phase Correction\n(radians)" class="Slide (strict)"("Visible"=TRUE) -> ()  [unwired: 2 in, 2 out]
              }
            }
            n143 = call "IMAQ Histograph"("Image"=w311) -> ("Histogram Graph"=w322:T22)  [unwired: 7 in, 3 out]
            n144 = property on="Histogram" class="WFGraph (strict)"("Value"=w322) -> ()  [unwired: 2 in, 2 out]
          }
          frame "None", Default {
            n145 = case shown="\"Imaging Galvo\"" w381 {
              tunnel: [w390 w420 w505 w594] -> w380
              tunnel: w379 -> [w390 w419 w504 w603]
              tunnel: w378 -> [w389 w401 w503 w600]
              tunnel: w377 -> [w388 w416 w502 w599]
              tunnel: [w388 w417 w501 w596] -> w376
              tunnel: [w389 w418 w500 w595] -> w375
              tunnel: w374 -> [w387 w415 w496 w601]
              tunnel: [w387 w414 w497 w597] -> w373
              tunnel: [w386 w413 w498 w598] -> w372
              tunnel: w371 -> [w386 w412 w499 w602]
              tunnel: [w385 w410 w494 w591] -> w370
              tunnel: w369 -> [w385 w411 w495 w592]
              tunnel: w368 -> [_ w409 w482 w580]
              tunnel: [w384 w408 w493 w590] -> w367
              tunnel: w366 -> [w384 w407 w492 w589]
              tunnel: w365 -> [w383 w406 w491 w588]
              tunnel: [w383 w405 w490 w587] -> w364
              tunnel: w363 -> [_ w404 w489 _]
              tunnel: [w382 w403 w488 w586] -> w362
              tunnel: w361 -> [w382 w402 w487 w585]
              frame "SciScan Disconnected", Default {
              }
              frame "Uncaging Galvo" {
                n146 = call "GFGTranslator__WRAPPER.vi"("GFGTranslator Datatype"=GFGTranslator_Datatype."Numeric", "GFG Translator Action"=GFGTranslator_Action."Get", "GFG Variable Name"="MAIN.Image.panels.") -> ("Numeric_Output"=w397:dbl, "Status Output"=w396:T20)  [unwired: 3 in, 4 out]
                n147 = To Unsigned Long Integer(number=w397) -> (unsigned 32bit integer=w395:u32)
                n148 = Increment(x=w395) -> (x+1=w392:u32)
                n149 = In Range and Coerce(upper limit=u32 4, x=w392, lower limit=u32 1) -> (coerced(x)=w391:u32)  [unwired: 1 out]
                n150 = case shown="\"Success\"" w396 {
                  tunnel: w391 -> [w447 _]
                  tunnel: [w453 w481] -> w420
                  tunnel: w419 -> [_ w481]
                  tunnel: w401 -> [w433 w480]
                  tunnel: [w435 w480] -> w418
                  tunnel: [w424 w479] -> w417
                  tunnel: w416 -> [w432 w479]
                  tunnel: w415 -> [w452 w478]
                  tunnel: [w452 w478] -> w414
                  tunnel: [w421 w477] -> w413
                  tunnel: w412 -> [w422 w477]
                  tunnel: w411 -> [w451 w476]
                  tunnel: [w451 w476] -> w410
                  tunnel: w409 -> [_ _]
                  tunnel: [w426 w475] -> w408
                  tunnel: w407 -> [w428 w475]
                  tunnel: w406 -> [w449 w474]
                  tunnel: [w448 w474] -> w405
                  tunnel: w404 -> [_ _]
                  tunnel: [w445 w473] -> w403
                  tunnel: w402 -> [w445 w473]
                  frame "Success" {
                    # "Has  I Path Image been cleared?"
                    # "Has Imaging Path image been cleared?"
                    n151 = property on="Uncaging Histogram" class="Clust (strict)"() -> ("Value"=w446:T7)  [unwired: 2 in, 2 out]
                    n152 = Number To Decimal String(number=w447) -> (decimal integer string=w455:string)  [unwired: 1 in]
                    n153 = Concatenate Strings("Channel " ("GFG Variable Name"), w455, " large" ("string")) -> (w453:string)
                    n154 = property on="Uncaging Histogram" class="Clust (strict)"("Val(Sgnl)"=w446) -> ()  [unwired: 2 in, 2 out]
                    n155 = call "GFGTranslator__WRAPPER.vi"("GFGTranslator Datatype"=GFGTranslator_Datatype."Get_Variant", "GFG Translator Action"=GFGTranslator_Action."Get", "GFG Variable Name"=w453) -> ("Variant_Output"=w439:variant)  [unwired: 3 in, 5 out]
                    n156 = Variant To Data(type=T6 refnum ("New Image"), Variant=w439) -> (data=w434:T6)  [unwired: 1 in, 1 out]
                    n157 = call "Check for change in Image Sizes.vi"("Other optical path [Current ImRef]"=w432, "Current Optical Path [New ImRef]"=w434, "Current Optical Path [Current ImRef]"=w433) -> ("Other Optical Path [New ImRef] OUT"=w424:T6, "Current Optical Path [New ImRef] OUT"=w431:T6)  [unwired: 7 in]
                    n158 = call "IMAQ GetImageSize"("Image"=w424) -> ("Y Resolution"=w430:i32)  [unwired: 3 in, 2 out]
                    n159 = Less Or Equal To 0?(x=w430) -> (x <= 0?=w429:bool)
                    n160 = call "IMAQ Copy"("Image Dst"=w433, "Image Src"=w431) -> ("Image Dst Out"=w435:T6)  [unwired: 4 in, 1 out]
                    n161 = Select(t=CalibrationType."None", s=w429, f=w428) -> (s? t:f=w426:T14)
                    n162 = case shown="\"None\", Default" w426 {
                      tunnel: [_ ", Imaging Galvo" ("regular expression") ", Imaging Reso" ("regular expression")] -> w450
                      frame "None", Default {
                      }
                      frame "ImagingGalvoCalibration" {
                      }
                      frame "ImagingResoCalibration" {
                      }
                    }
                    n163 = call "IMAQ GetImageSize"("Image"=w424) -> ("Y Resolution"=w425:i32)  [unwired: 3 in, 2 out]
                    n164 = call "IMAQ GetImageSize"("Image"=w431) -> ("Y Resolution"=w442:i32)  [unwired: 3 in, 2 out]
                    n165 = Less Or Equal To 0?(x=w425) -> (x <= 0?=w423:bool)
                    n166 = Less Or Equal To 0?(x=w442) -> (x <= 0?=w437:bool)
                    n167 = case "Clear Scaled image if IPath image has been cleared" shown="True" w423 {
                      tunnel: w422 -> [w457 w460]
                      tunnel: [w457 w458] -> w421
                      frame False {
                      }
                      frame True {
                        w459 = 0 ("X Resolution")
                        n168 = call "IMAQ SetImageSize"("Y Resolution"=w459, "X Resolution"=w459, "Image"=w460) -> ("Image Out"=w458:T6)  [unwired: 2 in, 1 out]
                      }
                    }
                    n169 = Select(t="", s=w437, f="PhotoStim Galvo" ("regular expression")) -> (s? t:f=w436:string)
                    n170 = case shown="False" w437 {
                      tunnel: w450 -> [w467 _]
                      tunnel: w449 -> [w466 w470]
                      tunnel: [w464 w470] -> w448
                      tunnel: w436 -> [w463 _]
                      frame False {
                        n171 = Concatenate Strings(w463, w467) -> (w465:string)
                        n172 = Replace Array Subset(array=w466, new element=w465, index (row)=3, index (col)=1 ("disabled index (col)")) -> (w464:string[][])
                        n173 = call "FGV_Calibration_KeyParams.vi"("Action"=FGV_CalibrationKeyParams_Actions."Grab From SciScan and Store", "System Type"="Stimulation Path Galvo") -> ()  [unwired: 4 in, 6 out]
                      }
                      frame True {
                        # "Empty image - do nothing!"
                      }
                    }
                  }
                  frame Default {
                  }
                }
              }
              frame "Imaging Galvo" {
                n174 = call "GFGTranslator__WRAPPER.vi"("GFGTranslator Datatype"=GFGTranslator_Datatype."Numeric", "GFG Translator Action"=GFGTranslator_Action."Get", "GFG Variable Name"="MAIN.Image.panels.") -> ("Numeric_Output"=w508:dbl, "Status Output"=w507:T20)  [unwired: 3 in, 4 out]
                n175 = To Unsigned Long Integer(number=w508) -> (unsigned 32bit integer=w506:u32)
                n176 = Increment(x=w506) -> (x+1=w486:u32)
                n177 = In Range and Coerce(upper limit=u32 4, x=w486, lower limit=u32 1) -> (coerced(x)=w483:u32)  [unwired: 1 out]
                n178 = case shown="\"Success\"" w507 {
                  tunnel: w483 -> [w541 _]
                  tunnel: [w546 w579] -> w505
                  tunnel: w504 -> [_ w579]
                  tunnel: w503 -> [w517 w577]
                  tunnel: w502 -> [w519 w578]
                  tunnel: [w522 w578] -> w501
                  tunnel: [w514 w577] -> w500
                  tunnel: w499 -> [w545 w575]
                  tunnel: [w545 w575] -> w498
                  tunnel: [w512 w576] -> w497
                  tunnel: w496 -> [w513 w576]
                  tunnel: w495 -> [w544 w574]
                  tunnel: [w544 w574] -> w494
                  tunnel: [w527 w573] -> w493
                  tunnel: w492 -> [w528 w573]
                  tunnel: w491 -> [w543 w572]
                  tunnel: [w542 w572] -> w490
                  tunnel: w489 -> [_ _]
                  tunnel: [w521 w571] -> w488
                  tunnel: w487 -> [w521 w571]
                  tunnel: w482 -> [w523 _]
                  frame "Success" {
                    # "Flip for Galvo Disabled!!!"
                    # "Has  SPath Image been cleared?"
                    # "Flip for Galvo"
                    n179 = property on="Imaging Path Histogram" class="Clust (strict)"() -> ("Value"=w540:T8)  [unwired: 2 in, 2 out]
                    n180 = Number To Decimal String(number=w541) -> (decimal integer string=w548:string)  [unwired: 1 in]
                    n181 = call "IMAQ GetImageSize"("Image"=w517) -> ("Y Resolution"=w536:i32)  [unwired: 3 in, 2 out]
                    n182 = property class="Bool (strict)"(reference=w523, "Value"=T11 FALSE) -> (reference out=w524:refnum<vi>, error out=w525:errorcluster)  [unwired: 1 in]
                    n183 = Less Or Equal To 0?(x=w536) -> (x <= 0?=w535:bool)
                    n184 = Concatenate Strings("Channel " ("GFG Variable Name"), w548, " large" ("string")) -> (w546:string)
                    n185 = Select(t="", s=w535, f="PhotoStim Galvo, " ("regular expression")) -> (s? t:f=w537:string)
                    n186 = Close Reference(reference=w524, error in (no error)=w525) -> ()  [unwired: 1 out]
                    n187 = property on="Imaging Path Histogram" class="Clust (strict)"("Val(Sgnl)"=w540) -> ()  [unwired: 2 in, 2 out]
                    n188 = call "GFGTranslator__WRAPPER.vi"("GFGTranslator Datatype"=GFGTranslator_Datatype."Get_Variant", "GFG Translator Action"=GFGTranslator_Action."Get", "GFG Variable Name"=w546) -> ("Variant_Output"=w531:variant)  [unwired: 3 in, 5 out]
                    n189 = Variant To Data(type=T6 refnum ("New Image"), Variant=w531) -> (data=w520:T6)  [unwired: 1 in, 1 out]
                    n190 = call "Check for change in Image Sizes.vi"("Other optical path [Current ImRef]"=w517, "Current Optical Path [New ImRef]"=w520, "Current Optical Path [Current ImRef]"=w519) -> ("Other Optical Path [New ImRef] OUT"=w514:T6, "Current Optical Path [New ImRef] OUT"=w518:T6)  [unwired: 7 in]
                    n191 = call "IMAQ GetImageSize"("Image"=w518) -> ("Y Resolution"=w530:i32)  [unwired: 3 in, 2 out]
                    n192 = call "IMAQ GetImageSize"("Image"=w514) -> ("Y Resolution"=w516:i32)  [unwired: 3 in, 2 out]
                    n193 = Less Or Equal To 0?(x=w530) -> (x <= 0?=w529:bool)
                    n194 = Less Or Equal To 0?(x=w516) -> (x <= 0?=w515:bool)
                    n195 = case "Clear Scaled image if SPath image has been cleared" shown="True" w515 {
                      tunnel: w513 -> [w550 w553]
                      tunnel: [w550 w551] -> w512
                      frame False {
                      }
                      frame True {
                        w552 = 0 ("X Resolution")
                        n196 = call "IMAQ SetImageSize"("Y Resolution"=w552, "X Resolution"=w552, "Image"=w553) -> ("Image Out"=w551:T6)  [unwired: 2 in, 1 out]
                      }
                    }
                    n197 = call "IMAQ Copy"("Image Dst"=w519, "Image Src"=w518) -> ("Image Dst Out"=w522:T6)  [unwired: 4 in, 1 out]
                    n198 = case shown="False" w529 {
                      tunnel: w543 -> [w561 w570]
                      tunnel: [w559 w570] -> w542
                      tunnel: w537 -> [w558 _]
                      tunnel: w528 -> [_ w566]
                      tunnel: [CalibrationType."ImagingGalvoCalibration" ("Curretn Calibration Type") w565] -> w527
                      frame False {
                        n199 = Concatenate Strings(w558, "Imaging Galvo" ("regular expression")) -> (w562:string)
                        n200 = property on="Sinusoidal Phase Correction\n(radians)" class="Slide (strict)"("Visible"=FALSE) -> ()  [unwired: 2 in, 2 out]
                        n201 = call "FGV_Calibration_KeyParams.vi"("Action"=FGV_CalibrationKeyParams_Actions."Grab From SciScan and Store", "System Type"="Imaging Path Galvo") -> ()  [unwired: 4 in, 6 out]
                        n202 = Replace Array Subset(array=w561, new element=w562, index (row)=3, index (col)=1 ("disabled index (col)")) -> (w559:string[][])
                      }
                      frame True {
                        # "clear Calibration type if Galvo image cleared"
                        # "Do nothing! - No valid image"
                        n203 = Equal?(x=CalibrationType."ImagingGalvoCalibration" ("Curretn Calibration Type"), y=w566) -> (x = y?=w568:bool)
                        n204 = Select(t=CalibrationType."None" ("Curretn Calibration Type"), s=w568, f=w566) -> (s? t:f=w565:T14)
                      }
                    }
                  }
                  frame Default {
                  }
                }
              }
              frame "Imaging Reso" {
                n205 = call "GFGTranslator__WRAPPER.vi"("GFGTranslator Datatype"=GFGTranslator_Datatype."Numeric", "GFG Translator Action"=GFGTranslator_Action."Get", "GFG Variable Name"="MAIN.Image.panels.reso.") -> ("Numeric_Output"=w605:dbl, "Status Output"=w593:T20)  [unwired: 3 in, 4 out]
                n206 = To Unsigned Long Integer(number=w605) -> (unsigned 32bit integer=w604:u32)
                n207 = Increment(x=w604) -> (x+1=w582:u32)
                n208 = In Range and Coerce(upper limit=u32 4, x=w582, lower limit=u32 1) -> (coerced(x)=w581:u32)  [unwired: 1 out]
                n209 = case shown="\"Success\"" w593 {
                  tunnel: w581 -> [w639 _]
                  tunnel: [w640 w677] -> w594
                  tunnel: w603 -> [_ w677]
                  tunnel: w600 -> [w615 w675]
                  tunnel: w599 -> [w617 w676]
                  tunnel: [w621 w676] -> w596
                  tunnel: [w612 w675] -> w595
                  tunnel: w602 -> [w609 w673]
                  tunnel: [w609 w673] -> w598
                  tunnel: [w610 w674] -> w597
                  tunnel: w601 -> [w611 w674]
                  tunnel: w592 -> [w644 w672]
                  tunnel: [w644 w672] -> w591
                  tunnel: [w626 w671] -> w590
                  tunnel: w589 -> [w627 w671]
                  tunnel: w588 -> [w643 w670]
                  tunnel: [w642 w670] -> w587
                  tunnel: [w619 w669] -> w586
                  tunnel: w585 -> [_ w669]
                  tunnel: w580 -> [w625 _]
                  frame "Success" {
                    # "Has  SPath Image been cleared?"
                    # "No flip for Reso"
                    n210 = property on="Imaging Path Histogram" class="Clust (strict)"() -> ("Value"=w641:T8)  [unwired: 2 in, 2 out]
                    n211 = Number To Decimal String(number=w639) -> (decimal integer string=w646:string)  [unwired: 1 in]
                    n212 = call "IMAQ GetImageSize"("Image"=w615) -> ("Y Resolution"=w632:i32)  [unwired: 3 in, 2 out]
                    n213 = property class="Bool (strict)"(reference=w625, "Value"=T11 FALSE) -> (reference out=w622:refnum<vi>, error out=w623:errorcluster)  [unwired: 1 in]
                    n214 = Less Or Equal To 0?(x=w632) -> (x <= 0?=w631:bool)
                    n215 = Concatenate Strings("Channel " ("GFG Variable Name"), w646, " large" ("string")) -> (w640:string)
                    n216 = Close Reference(reference=w622, error in (no error)=w623) -> ()  [unwired: 1 out]
                    n217 = call "GFGTranslator__WRAPPER.vi"("GFGTranslator Datatype"=GFGTranslator_Datatype."Get_Variant", "GFG Translator Action"=GFGTranslator_Action."Get", "GFG Variable Name"=w640) -> ("Variant_Output"=w635:variant)  [unwired: 3 in, 5 out]
                    n218 = Select(t="", s=w631, f="PhotoStim Galvo, " ("regular expression")) -> (s? t:f=w628:string)
                    n219 = property on="Imaging Path Histogram" class="Clust (strict)"("Val(Sgnl)"=w641) -> ()  [unwired: 2 in, 2 out]
                    n220 = Variant To Data(type=T6 refnum ("New Image"), Variant=w635) -> (data=w618:T6)  [unwired: 1 in, 1 out]
                    n221 = call "Check for change in Image Sizes.vi"("Other optical path [Current ImRef]"=w615, "Current Optical Path [New ImRef]"=w618, "Current Optical Path [Current ImRef]"=w617) -> ("Other Optical Path [New ImRef] OUT"=w612:T6, "Current Optical Path [New ImRef] OUT"=w616:T6)  [unwired: 7 in]
                    n222 = call "IMAQ GetImageSize"("Image"=w612) -> ("Y Resolution"=w614:i32)  [unwired: 3 in, 2 out]
                    n223 = Less Or Equal To 0?(x=w614) -> (x <= 0?=w613:bool)
                    n224 = case "Clear Scaled image if SPath image has been cleared" shown="True" w613 {
                      tunnel: w611 -> [w648 w651]
                      tunnel: [w648 w649] -> w610
                      frame False {
                      }
                      frame True {
                        w650 = 0 ("X Resolution")
                        n225 = call "IMAQ SetImageSize"("Y Resolution"=w650, "X Resolution"=w650, "Image"=w651) -> ("Image Out"=w649:T6)  [unwired: 2 in, 1 out]
                      }
                    }
                    n226 = call "IMAQ GetImageSize"("Image"=w616) -> ("Y Resolution"=w630:i32)  [unwired: 3 in, 2 out]
                    n227 = Less Or Equal To 0?(x=w630) -> (x <= 0?=w629:bool)
                    n228 = call "IMAQ Copy"("Image Dst"=w617, "Image Src"=w616) -> ("Image Dst Out"=w621:T6)  [unwired: 4 in, 1 out]
                    n229 = case shown="True" w629 {
                      tunnel: w643 -> [w658 w668]
                      tunnel: [w657 w668] -> w642
                      tunnel: w628 -> [w656 _]
                      tunnel: w627 -> [_ w664]
                      tunnel: [CalibrationType."ImagingResoCalibration" ("Curretn Calibration Type") w663] -> w626
                      frame False {
                        n230 = Concatenate Strings(w656, "Imaging Reso" ("regular expression")) -> (w660:string)
                        n231 = Replace Array Subset(array=w658, new element=w660, index (row)=3, index (col)=1 ("disabled index (col)")) -> (w657:string[][])
                        n232 = call "FGV_Calibration_KeyParams.vi"("Action"=FGV_CalibrationKeyParams_Actions."Grab From SciScan and Store", "System Type"="Imaging Path Reso") -> ()  [unwired: 4 in, 6 out]
                        n233 = property on="Sinusoidal Phase Correction\n(radians)" class="Slide (strict)"("Visible"=TRUE) -> ()  [unwired: 2 in, 2 out]
                      }
                      frame True {
                        # "clear Calibration type if Reso image cleared"
                        # "Do nothing! - No valid image"
                        # "Do nothing! - No valid image"
                        n234 = Equal?(x=CalibrationType."ImagingResoCalibration" ("Curretn Calibration Type"), y=w664) -> (x = y?=w666:bool)
                        n235 = Select(t=CalibrationType."None" ("Curretn Calibration Type"), s=w666, f=w664) -> (s? t:f=w663:T14)
                      }
                    }
                    n236 = call "GFGnumericGet.vi"("Variable Name in"="Start.Delay") -> ("Numeric"=w619:dbl)  [unwired: 8 in, 2 out]
                  }
                  frame Default {
                  }
                }
              }
            }
            n237 = global write "Global_CalibrationSimulation.vi" "Simulation?"(FALSE ("Simulation?")) -> ()
          }
        }
      }
      event Value Change {
        n238 = event-data() -> ()  [unwired: 1 in, 1 out]
        n239 = call "IMAQ GetImageSize"("Image"=w685) -> ("Y Resolution"=w686:i32)  [unwired: 3 in, 2 out]
        n240 = call "IMAQ GetImageSize"("Image"=w683) -> ("Y Resolution"=w684:i32)  [unwired: 3 in, 2 out]
        n241 = Less Or Equal To 0?(x=w686) -> (x <= 0?=w682:bool)
        n242 = Less Or Equal To 0?(x=w684) -> (x <= 0?=w681:bool)
        n243 = Or(x=w682, y=w681) -> (x .or. y?=w680:bool)
        n244 = case shown="False" w680 {
          tunnel: w679 -> [w697 _]
          tunnel: w678 -> [w696 _]
          frame False {
            n245 = case shown="\"ImagingResoCalibration\"" w697 {
              tunnel: w696 -> [_ w714 w735]
              frame Default {
              }
              frame "ImagingGalvoCalibration" {
                w708 = "Galvo Calibration" ("Calibration Type")
                n246 = Index Array(array=w714, index=0) -> (element=w712:path)
                n247 = call "CalibrationFileIO.vi"("Calibration Type"=w708, "CalibrationFileIO_command"=enum16{"WriteSettings", "ReadSettings"}."ReadSettings", "configuration file path"=w712) -> ("Common Parameters OUT"=w711:T21)  [unwired: 6 in, 2 out]
                n248 = call "Calibration_Estimate X and Y Zoom voltages.vi"("System Type"=w708) -> ("Y.ZOOM_estimated"=w706:dbl, "X.ZOOM_estimated"=w707:dbl)  [unwired: 9 in]
                n249 = Unbundle By Name(w711) -> ("X.ZOOM.Compensation"=w710:dbl, "Y.ZOOM.Compensation"=w709:dbl)
                n250 = Multiply(x=w707, y=w710) -> (x*y=w703:dbl)
                n251 = Multiply(x=w706, y=w709) -> (x*y=w699:dbl)
                n252 = In Range and Coerce(upper limit=20.0, x=w703, lower limit=1.0) -> (coerced(x)=w702:dbl)  [unwired: 1 out]
                n253 = In Range and Coerce(upper limit=20.0, x=w699, lower limit=1.0) -> (coerced(x)=w698:dbl)  [unwired: 1 out]
                n254 = Bundle By Name(cluster=cluster{"X.Zoom":dbl, "Y.Zoom":dbl} {"X.Zoom"=0.0, "Y.Zoom"=0.0} ("Value (Signaling)"), "X.Zoom"=w702, "Y.Zoom"=w698) -> (w716:cluster{"X.Zoom":dbl, "Y.Zoom":dbl})
                n255 = property on="Linear Zoom" class="Clust (strict)"("Val(Sgnl)"=w716) -> ()  [unwired: 2 in, 2 out]
              }
              frame "ImagingResoCalibration" {
                w726 = "Reso Calibration" ("Calibration Type")
                n256 = Index Array(array=w735, index=1) -> (element=w733:path)
                n257 = call "CalibrationFileIO.vi"("Calibration Type"=w726, "CalibrationFileIO_command"=enum16{"WriteSettings", "ReadSettings"}."ReadSettings", "configuration file path"=w733) -> ("Common Parameters OUT"=w732:T21)  [unwired: 6 in, 2 out]
                n258 = call "Calibration_Estimate X and Y Zoom voltages.vi"("System Type"=w726) -> ("Y.ZOOM_estimated"=w727:dbl, "X.ZOOM_estimated"=w728:dbl)  [unwired: 9 in]
                n259 = Unbundle By Name(w732) -> ("X.ZOOM.Compensation"=w731:dbl, "Y.ZOOM.Compensation"=w730:dbl, "Reso_Phase.Correction"=w729:dbl)
                n260 = Multiply(x=w728, y=w731) -> (x*y=w723:dbl)
                n261 = Multiply(x=w727, y=w730) -> (x*y=w719:dbl)
                n262 = In Range and Coerce(upper limit=20.0, x=w723, lower limit=1.0) -> (coerced(x)=w722:dbl)  [unwired: 1 out]
                n263 = In Range and Coerce(upper limit=20.0, x=w719, lower limit=1.0) -> (coerced(x)=w718:dbl)  [unwired: 1 out]
                n264 = Bundle By Name(cluster=cluster{"X.Zoom":dbl, "Y.Zoom":dbl} {"X.Zoom"=0.0, "Y.Zoom"=0.0} ("Value (Signaling)"), "X.Zoom"=w722, "Y.Zoom"=w718) -> (w737:cluster{"X.Zoom":dbl, "Y.Zoom":dbl})
                n265 = property on="Sinusoidal Phase Correction\n(radians)" class="Slide (strict)"("Value"=w729) -> ()  [unwired: 2 in, 2 out]
                n266 = property on="Linear Zoom" class="Clust (strict)"("Val(Sgnl)"=w737) -> ()  [unwired: 2 in, 2 out]
              }
            }
          }
          frame True {
            n267 = One Button Dialog(message="Auto-Calibration requires images from both optical paths!\nPlease acquire both the images and try again...\n") -> ()  [unwired: 1 in, 1 out]
          }
        }
      }
      event "reset zoom_Calibration_UI": Value Change {
        n268 = event-data() -> ()  [unwired: 1 in, 1 out]
        n269 = property on="Source Images" class="TabCtl (strict)"() -> ("Value"=w744:T5)  [unwired: 2 in, 2 out]
        n270 = property class="ImageControl"(reference=w740, "Zoom to Fit Mode"=TRUE) -> ()  [unwired: 1 in, 2 out]
        n271 = case shown="\"Stimulation Path Image\", Default" w744 {
          tunnel: w743 -> [_ w760]
          tunnel: w742 -> [w757 _]
          frame "Stimulation Path Image", Default {
            n272 = property class="ImageControl"(reference=w757, "Zoom to Fit Mode"=TRUE) -> ()  [unwired: 1 in, 2 out]
          }
          frame "Imaging Path Image" {
            n273 = property class="ImageControl"(reference=w760, "Zoom to Fit Mode"=TRUE) -> ()  [unwired: 1 in, 2 out]
          }
        }
      }
      event "Calibration File I/O.Save Calibration": Value Change {
        # "Check for equal size"
        n274 = event-data() -> ()  [unwired: 1 in, 1 out]
        n275 = call "IMAQ GetImageSize"("Image"=w772) -> ("Y Resolution"=w764:i32, "X Resolution"=w765:i32)  [unwired: 3 in, 1 out]
        n276 = call "IMAQ GetImageSize"("Image"=w771) -> ("Y Resolution"=w769:i32, "X Resolution"=w770:i32)  [unwired: 3 in, 1 out]
        n277 = Greater Than 0?(x=w765) -> (x > 0?=w762:bool)
        n278 = Greater Than 0?(x=w764) -> (x > 0?=w763:bool)
        n279 = Equal?(x=w765, y=w770) -> (x = y?=w768:bool)
        n280 = Equal?(x=w764, y=w769) -> (x = y?=w767:bool)
        n281 = Compound Arithmetic op=AND(w762, w763, w768, w767) -> (w766:bool)
        n282 = case shown="True" w766 {
          tunnel: w778 -> [_ w794]
          tunnel: w777 -> [_ w793]
          tunnel: w776 -> [_ w792]
          tunnel: w775 -> [w787 w791]
          tunnel: [w787 w788] -> w774
          tunnel: w773 -> [_ w790]
          tunnel: w761 -> [_ w789]
          frame False {
            w786 = "Cannot Save Calibration! \nPlease try again with two equally sized images."  # GUI message when image size does not fit
            n283 = One Button Dialog(message=w786) -> ()  [unwired: 1 in, 1 out]
          }
          frame True {
            n284 = case shown="\"ImagingGalvoCalibration\"" w794 {
              tunnel: w793 -> [_ w834 w869]
              tunnel: w792 -> [_ w825 w860]
              tunnel: w791 -> [w799 w813 w850]
              tunnel: [w799 w812 w846] -> w788
              tunnel: w790 -> [_ _ _]
              tunnel: w789 -> [_ w810 w845]
              frame "None", Default {
                n285 = One Button Dialog(message="Either Galvo or Reso image needs to be selected") -> ()  [unwired: 1 in, 1 out]
              }
              frame "ImagingGalvoCalibration" {
                w801 = 0.0  # No phase correction for Galvo!
                w809 = 0 ("index")
                n286 = property on="Linear Zoom" class="Clust (strict)"() -> ("Value"=w807:cluster{"X.Zoom":dbl, "Y.Zoom":dbl})  [unwired: 2 in, 2 out]
                n287 = Get Date/Time In Seconds() -> (seconds since 1Jan1904=w819:timestamp)
                n288 = property on="Non Linear Stretch" class="Clust (strict)"() -> ("Value"=w806:T10)  [unwired: 2 in, 2 out]
                n289 = property on="X-Offset (Pixels)" class="Slide (strict)"() -> ("Value"=w804:i32)  [unwired: 2 in, 2 out]
                n290 = property on="Y-Offset (Pixels)" class="Slide (strict)"() -> ("Value"=w805:i32)  [unwired: 2 in, 2 out]
                n291 = property on="Sinusoidal Phase Correction\n(radians)" class="Slide (strict)" props=["Value"]() -> ()  [unwired: 2 in, 3 out]
                n292 = Format Date/Time String(seconds (now)=w819) -> (date/time string=w811:string)  [unwired: 2 in]
                n293 = Index Array(array=w834, index=w809) -> (element=w832:path)
                n294 = Index Array "Calibration Type"(array=w810, index=w809) -> (element=w808:string)
                n295 = Unbundle By Name(w806) -> ("Phase Offset (2-35%)"=w827:dbl, "Magnitude (0-1)"=w826:dbl)
                n296 = property class="Bool (strict)"(reference=w825) -> ("Value"=w824:T11)  [unwired: 1 in, 2 out]
                n297 = Unbundle By Name(w807) -> ("X.Zoom"=w829:dbl, "Y.Zoom"=w828:dbl)
                n298 = Bundle By Name(cluster=T21 {"X.ZOOM.Compensation"=1.0, "Y.ZOOM.Compensation"=1.0, "Reso_Phase.Correction"=0.0} ("Common Parameters IN"), "Reso_Phase.Correction"=w801) -> (w802:T21)
                n299 = local read "X-Pixel Mapping"() -> (w822:i16[])
                n300 = local read "Y-Pixel Mapping"() -> (w821:i16[])
                n301 = Bundle By Name(cluster=T17 {"General_Parameters"={"SystemType"="", "Date/Time String"=""}, "Corection Parameters"={"X-Offset"=0, "Y-Offset"=0, "X-Zoom"=0.0, "Y-Zoom"=0.0, "PhaseOffset"=0.0, "Magnification"=0.0, "Flip"=FALSE}, "GFG Params(Numeric)"=[]} ("Calibration paramaters_IN"), "General_Parameters.SystemType"="Galvo", "General_Parameters.Date/Time String"=w811, "Corection Parameters.X-Offset"=w804, "Corection Parameters.Y-Offset"=w805, "Corection Parameters.X-Zoom"=w829, "Corection Parameters.Y-Zoom"=w828, "Corection Parameters.PhaseOffset"=w827, "Corection Parameters.Magnification"=w826, "Corection Parameters.Flip"=w824) -> (w823:T17)
                n302 = Bundle("X-Pixel Mapping"=w822, "Y-Pixel Mapping"=w821) -> (w820:T24)  [unwired: 1 in]
                n303 = call "CalibrationFileIO.vi"("Calibration Type"=w808, "CalibrationFileIO_command"=enum16{"WriteSettings", "ReadSettings"}."WriteSettings", "Pixel Mapping to Write"=w820, "Common Parameters IN"=w802, "Calibration paramaters_IN"=w823, "configuration file path"=w832) -> ("Calibration paramaters_OUT"=w816:T17)  [unwired: 3 in, 2 out]
                n304 = Replace Array Subset(array=w813, new element=w811, index (row)=1, index (col)=1 ("disabled index (col)")) -> (w812:string[][])
                n305 = Concatenate Strings("Galvo calibration has been updated!\nTimestamp: " ("General_Parameters.SystemType"), w811) -> (w817:string)
                n306 = flat-sequence {
                  tunnel: w817 -> [w835]
                  tunnel: w816 -> [_]
                  frame #0 {
                    n307 = One Button Dialog(message=w835) -> ()  [unwired: 1 in, 1 out]
                  }
                }
              }
              frame "ImagingResoCalibration" {
                w844 = 1 ("index")
                n308 = Get Date/Time In Seconds() -> (seconds since 1Jan1904=w854:timestamp)
                n309 = property on="Linear Zoom" class="Clust (strict)"() -> ("Value"=w842:cluster{"X.Zoom":dbl, "Y.Zoom":dbl})  [unwired: 2 in, 2 out]
                n310 = property on="Y-Offset (Pixels)" class="Slide (strict)"() -> ("Value"=w839:i32)  [unwired: 2 in, 2 out]
                n311 = property on="X-Offset (Pixels)" class="Slide (strict)"() -> ("Value"=w840:i32)  [unwired: 2 in, 2 out]
                n312 = property on="Sinusoidal Phase Correction\n(radians)" class="Slide (strict)"() -> ("Value"=w837:dbl)  [unwired: 2 in, 2 out]
                n313 = property on="Non Linear Stretch" class="Clust (strict)"() -> ("Value"=w841:T10)  [unwired: 2 in, 2 out]
                n314 = Format Date/Time String(seconds (now)=w854) -> (date/time string=w847:string)  [unwired: 2 in]
                n315 = Index Array(array=w869, index=w844) -> (element=w867:path)
                n316 = Index Array "Calibration Type"(array=w845, index=w844) -> (element=w843:string)
                n317 = Bundle By Name(cluster=T21 {"X.ZOOM.Compensation"=1.0, "Y.ZOOM.Compensation"=1.0, "Reso_Phase.Correction"=0.0} ("Common Parameters IN"), "Reso_Phase.Correction"=w837) -> (w836:T21)
                n318 = property class="Bool (strict)"(reference=w860) -> ("Value"=w859:T11)  [unwired: 1 in, 2 out]
                n319 = Unbundle By Name(w842) -> ("X.Zoom"=w864:dbl, "Y.Zoom"=w863:dbl)
                n320 = Unbundle By Name(w841) -> ("Phase Offset (2-35%)"=w862:dbl, "Magnitude (0-1)"=w861:dbl)
                n321 = local read "X-Pixel Mapping"() -> (w857:i16[])
                n322 = local read "Y-Pixel Mapping"() -> (w856:i16[])
                n323 = Bundle By Name(cluster=T17 {"General_Parameters"={"SystemType"="", "Date/Time String"=""}, "Corection Parameters"={"X-Offset"=0, "Y-Offset"=0, "X-Zoom"=0.0, "Y-Zoom"=0.0, "PhaseOffset"=0.0, "Magnification"=0.0, "Flip"=FALSE}, "GFG Params(Numeric)"=[]} ("Calibration paramaters_IN"), "General_Parameters.SystemType"="Reso", "General_Parameters.Date/Time String"=w847, "Corection Parameters.X-Offset"=w840, "Corection Parameters.Y-Offset"=w839, "Corection Parameters.X-Zoom"=w864, "Corection Parameters.Y-Zoom"=w863, "Corection Parameters.PhaseOffset"=w862, "Corection Parameters.Magnification"=w861, "Corection Parameters.Flip"=w859) -> (w858:T17)
                n324 = Bundle("X-Pixel Mapping"=w857, "Y-Pixel Mapping"=w856) -> (w855:T24)  [unwired: 1 in]
                n325 = call "CalibrationFileIO.vi"("Calibration Type"=w843, "CalibrationFileIO_command"=enum16{"WriteSettings", "ReadSettings"}."WriteSettings", "Pixel Mapping to Write"=w855, "Common Parameters IN"=w836, "Calibration paramaters_IN"=w858, "configuration file path"=w867) -> ("Calibration paramaters_OUT"=w851:T17)  [unwired: 3 in, 2 out]
                n326 = Replace Array Subset(array=w850, new element=w847, index (row)=2, index (col)=1 ("disabled index (col)")) -> (w846:string[][])
                n327 = Concatenate Strings("Reso calibration has been updated!\nTimestamp: " ("General_Parameters.SystemType"), w847) -> (w852:string)
                n328 = flat-sequence {
                  tunnel: w852 -> [w870]
                  tunnel: w851 -> [_]
                  frame #0 {
                    n329 = One Button Dialog(message=w870) -> ()  [unwired: 1 in, 1 out]
                  }
                }
              }
            }
            n330 = flat-sequence {
              tunnel: w788 -> [_]
              frame #0 {
                # "Flag a Calibration Change!"
                n331 = call "GFGTranslator__WRAPPER.vi"("GFGTranslator Datatype"=GFGTranslator_Datatype."Boolean", "GFG Translator Action"=GFGTranslator_Action."Set", "Boolean_Input"=TRUE, "GFG Variable Name"="Flag_CalibrationChanged") -> ()  [unwired: 2 in, 6 out]
              }
            }
          }
        }
      }
      event Value Change {
        # "choose the max pixels (for the case if one image is empty!)"
        n332 = event-data() -> ()  [unwired: 1 in, 1 out]
        n333 = case shown="\"ImagingResoCalibration\"" w875 {
          tunnel: [0 ("x-1") 1 ("x-1")] -> w874
          frame "None", Default {
          }
          frame "ImagingResoCalibration" {
          }
        }
        n334 = call "IMAQ GetImageSize"("Image"=w885) -> ("Y Resolution"=w881:i32, "X Resolution"=w883:i32)  [unwired: 3 in, 1 out]
        n335 = call "IMAQ GetImageSize"("Image"=w884) -> ("Y Resolution"=w880:i32, "X Resolution"=w882:i32)  [unwired: 3 in, 1 out]
        n336 = Max & Min(x=w881, y=w880) -> (max(x,y)=w877:i32)  [unwired: 1 out]
        n337 = Max & Min(x=w883, y=w882) -> (max(x,y)=w878:i32)  [unwired: 1 out]
        n338 = Bundle By Name(cluster=cluster{"X Pixels":i32, "Y Pixels":i32} {"X Pixels"=0, "Y Pixels"=0} ("Current Image Pixels"), "X Pixels"=w878, "Y Pixels"=w877) -> (w876:cluster{"X Pixels":i32, "Y Pixels":i32})
        n339 = Index Array(array=w891, index=w874) -> (element=w890:path)
        n340 = Index Array(array=w887, index=w874) -> (element=w886:string)
        n341 = call "CalibrationFileIO.vi"("Current Image Pixels"=w876, "Calibration Type"=w886, "CalibrationFileIO_command"=enum16{"WriteSettings", "ReadSettings"}."ReadSettings", "configuration file path"=w890) -> ("Common Parameters OUT"=w873:T21, "Param Matches during a read"=w871:i32, "Calibration paramaters_OUT"=w889:T17)  [unwired: 5 in]
        n342 = Less Or Equal To 0?(x=w871) -> (x <= 0?=w872:bool)
        n343 = case shown="False" w872 {
          tunnel: w889 -> [w910 _]
          tunnel: w873 -> [w902 _]
          frame False {
            n344 = Unbundle By Name(w902) -> ("Reso_Phase.Correction"=w901:dbl)
            n345 = Unbundle By Name(w910) -> ("Corection Parameters.X-Offset"=w909:i32, "Corection Parameters.Y-Offset"=w908:i32)
            n346 = Unbundle By Name(w910) -> ("Corection Parameters.X-Zoom"=w905:dbl, "Corection Parameters.Y-Zoom"=w906:dbl)
            n347 = Unbundle By Name(w910) -> ("Corection Parameters.PhaseOffset"=w913:dbl, "Corection Parameters.Magnification"=w912:dbl)
            n348 = Unbundle By Name(w910) -> ("Corection Parameters.Flip"=w904:bool)
            n349 = Bundle By Name(cluster=T10 {"Phase Offset (2-35%)"=5.0, "Magnitude (0-1)"=0.0} ("Non Linear Stretch"), "Phase Offset (2-35%)"=w913, "Magnitude (0-1)"=w912) -> (w911:T10)
            n350 = Bundle By Name(cluster=cluster{"X.Zoom":dbl, "Y.Zoom":dbl} {"X.Zoom"=1.0, "Y.Zoom"=1.0} ("Linear Zoom"), "X.Zoom"=w905, "Y.Zoom"=w906) -> (w903:cluster{"X.Zoom":dbl, "Y.Zoom":dbl})
            n351 = property on="Non Linear Stretch" class="Clust (strict)"("Value"=w911) -> ()  [unwired: 2 in, 2 out]
            n352 = property on="X-Offset (Pixels)" class="Slide (strict)"("Value"=w909) -> ()  [unwired: 2 in, 2 out]
            n353 = property on="Y-Offset (Pixels)" class="Slide (strict)"("Value"=w908) -> ()  [unwired: 2 in, 2 out]
            n354 = property on="Linear Zoom" class="Clust (strict)"("Value"=w903) -> ()  [unwired: 2 in, 2 out]
            n355 = property on="Flip" class="Bool (strict)"("Val(Sgnl)"=w904) -> ()  [unwired: 2 in, 2 out]
            n356 = property on="Sinusoidal Phase Correction\n(radians)" class="Slide (strict)"("Value"=w901) -> ()  [unwired: 2 in, 2 out]
          }
          frame True {
            n357 = One Button Dialog(message="Could not find any matching calibrations!") -> ()  [unwired: 1 in, 1 out]
          }
        }
      }
      event Value Change {
        # "Trigger an Update"
        n358 = event-data() -> ()  [unwired: 1 in, 1 out]
      }
      event "Uncaging Histogram": Value Change {
        n359 = event-data() -> ("NewVal"=w947:T7)  [unwired: 1 in]
        n360 = property class="Bool (strict)"(reference=w934) -> (reference out=w935:refnum<vi>, error out=w936:errorcluster, "Value"=w937:T11)  [unwired: 1 in]
        n361 = control-ref of="Min Max (Red)"() -> (w944:refnum<vi>)
        n362 = Unbundle By Name(w947) -> ("auto scale\n      Red"=w945:bool)
        n363 = control-ref of="Histogram"() -> (w930:refnum<vi>)
        n364 = property class="Bool (strict)"(reference=w935, error in=w936, "Val(Sgnl)"=w937) -> ()  [unwired: 2 out]
        n365 = disable-structure shown="Enabled" {
          disable-tunnel: w946 -> [w979 w999]
          disable-tunnel: w945 -> [w977 w1007]
          disable-tunnel: w944 -> [w973 w1006]
          disable-tunnel: w941 -> [w972 w1003]
          disable-tunnel: w940 -> [w971 w1002]
          disable-tunnel: [w970 w1000] -> w939
          disable-tunnel: [w969 w1001] -> w938
          disable-tunnel: w931 -> [_ w1008]
          disable-tunnel: w930 -> [_ w998]
          frame Disabled {
            w976 = u32 14 items=["Default"=10, "Most Significant Bits"=11, "Full Dynamic"=12, "Downshift"=13, "Given Range"=14, "90% Dynamic"=15, "Given Percent Range"=16] ("16-bit Display Mapping:Conversion Method")
            # "Make values positive; starting from 0"
            # "Update Scaled Image"
            n366 = call "IMAQ ImageToArray"("Image"=w979) -> ("Image Pixels (I16)"=w953:i16[][])  [unwired: 3 in, 4 out]
            n367 = Array Max & Min(array=w953) -> (min value=w956:i16)  [unwired: 3 out]
            n368 = Less Than 0?(x=w956) -> (x < 0?=w957:bool)
            n369 = case shown="True" w957 {
              tunnel: w953 -> [w980 w984]
              tunnel: w956 -> [_ w983]
              tunnel: [w980 w981] -> w955
              frame False {
              }
              frame True {
                n370 = Negate(x=w983) -> (-x=w982:i16)
                n371 = Add(x=w984, y=w982) -> (x+y=w981:i16[][])
              }
            }
            n372 = Array Max & Min(array=w955) -> (max value=w974:i16, min value=w975:i16)  [unwired: 2 out]
            n373 = case shown="True" w977 {
              tunnel: w975 -> [_ w990]
              tunnel: w974 -> [_ w989]
              tunnel: w973 -> [w988 w992]
              tunnel: [w985 w989] -> w961
              tunnel: [w986 w990] -> w960
              frame False {
                n374 = property class="Slide (strict)"(reference=w988) -> ("Value"=w987:cluster{i16, i16})  [unwired: 1 in, 2 out]
                n375 = Unbundle(w987) -> (w986:i16, w985:i16)
              }
              frame True {
                n376 = Bundle(w990, w989) -> (w991:cluster{i16, i16})  [unwired: 1 in]
                n377 = property class="Slide (strict)"(reference=w992, "Value"=w991) -> ()  [unwired: 1 in, 2 out]
              }
            }
            n378 = Absolute Value(x=w960) -> (abs(x)=w963:i16)
            n379 = Absolute Value(x=w961) -> (abs(x)=w964:i16)
            n380 = In Range and Coerce(upper limit=w961, x=w955, lower limit=w960) -> (coerced(x)=w968:i16[][])  [unwired: 1 out]
            n381 = Max & Min(x=w964, y=w963) -> (max(x,y)=w962:i16)  [unwired: 1 out]
            n382 = control-ref of="Reference Image (From Uncaging Path)"() -> (w978:refnum<vi>)
            n383 = Divide(x=w968, y=w962) -> (x/y=w967:dbl[][])
            n384 = Multiply(x=w967, y=i16 255) -> (x*y=w965:dbl[][])
            n385 = To Unsigned Byte Integer(number=w965) -> (unsigned 8bit integer=w954:u8[][])
            n386 = Array Max & Min(array=w954) -> (max value=w959:u8, min value=w958:u8)  [unwired: 2 out]
            n387 = property class="ImageControl"(reference=w978, "16-bit Display Conversion Method"=w976, "16-bit Display Maximum Value"=w959, "16-bit Display Minimum Value"=w958) -> ()  [unwired: 1 in, 2 out]
            n388 = call "IMAQ ArrayToImage"("Image Pixels (U8)"=w954, "Image"=w972) -> ("Image Out"=w970:T6)  [unwired: 8 in, 1 out]
            n389 = call "IMAQ Copy"("Image Dst"=w971, "Image Src"=w970) -> ("Image Dst Out"=w969:T6)  [unwired: 4 in, 1 out]
          }
          frame Enabled {
            w1013 = u32 14 items=["Default"=10, "Most Significant Bits"=11, "Full Dynamic"=12, "Downshift"=13, "Given Range"=14, "90% Dynamic"=15, "Given Percent Range"=16] ("16-bit Display Mapping:Conversion Method")
            # "Copy normalised image to the image for transformation ('corrected image')"
            n390 = call "IMAQ ImageToArray"("Image"=w999) -> ("Image Pixels (I16)"=w1016:i16[][])  [unwired: 3 in, 4 out]
            n391 = call "IMAQ Histograph"("Image"=w999) -> ("Histogram Graph"=w997:T22)  [unwired: 7 in, 3 out]
            n392 = case shown="False" w1007 {
              tunnel: w1016 -> [w1043 w1057]
              tunnel: [w1036 w1047] -> w1015
              tunnel: [w1037 w1048] -> w1005
              tunnel: w1006 -> [w1044 w1055]
              tunnel: [w1043 w1057] -> w1004
              tunnel: w998 -> [w1039 w1052]
              tunnel: w997 -> [w1038 w1051]
              frame False {
                n393 = property class="Slide (strict)"(reference=w1044) -> (reference out=w1042:refnum<vi>, error out=w1046:errorcluster, "Value"=w1045:cluster{i16, i16})  [unwired: 1 in]
                n394 = Close Reference(reference=w1042, error in (no error)=w1046) -> ()  [unwired: 1 out]
                n395 = Unbundle(w1045) -> (w1037:i16, w1036:i16)
                n396 = property class="WFGraph (strict)"(reference=w1039, "Value"=w1038, "XScale.Minimum"=w1037, "XScale.Maximum"=w1036) -> (reference out=w1040:refnum<vi>, error out=w1041:errorcluster)  [unwired: 1 in]
                n397 = Close Reference(reference=w1040, error in (no error)=w1041) -> ()  [unwired: 1 out]
              }
              frame True {
                n398 = Array Max & Min(array=w1057) -> (max value=w1047:i16, min value=w1048:i16)  [unwired: 2 out]
                n399 = Bundle(w1048, w1047) -> (w1054:cluster{i16, i16})  [unwired: 1 in]
                n400 = property class="WFGraph (strict)"(reference=w1052, "Value"=w1051, "XScale.Minimum"=w1048, "XScale.Maximum"=w1047) -> (reference out=w1050:refnum<vi>, error out=w1049:errorcluster)  [unwired: 1 in]
                n401 = property class="Slide (strict)"(reference=w1055, "Value"=w1054, "Scale.Minimum"=w1048, "Scale.Maximum"=w1047) -> (reference out=w1053:refnum<vi>, error out=w1056:errorcluster)  [unwired: 1 in]
                n402 = Close Reference(reference=w1053, error in (no error)=w1056) -> ()  [unwired: 1 out]
                n403 = Close Reference(reference=w1050, error in (no error)=w1049) -> ()  [unwired: 1 out]
              }
            }
            n404 = To Long Integer(number=w1015) -> (32bit integer=w995:i32)
            n405 = To Long Integer(number=w1005) -> (32bit integer=w994:i32)
            n406 = To Long Integer(number=w1004) -> (32bit integer=w993:i32[][])
            n407 = Subtract "Data range"(x=w995, y=w994) -> (x-y=w1014:i32)
            n408 = disable-structure shown="Enabled" {
              disable-tunnel: w1014 -> [w1022 w1033]
              disable-tunnel: w993 -> [w1018 w1028]
              disable-tunnel: [w1017 w1031] -> w996
              frame Disabled {
                # "Make values positive; start from 0"
                # "compress data (lossy)"
                n409 = Array Max & Min(array=w1018) -> (min value=w1024:i32)  [unwired: 3 out]
                n410 = Negate(x=w1024) -> (-x=w1023:i32)
                n411 = Add(x=w1018, y=w1023) -> (x+y=w1025:i32[][])
                n412 = Divide(x=w1025, y=w1022) -> (x/y=w1021:dbl[][])
                n413 = Multiply(x=w1021, y=255.0 ("Numeric")) -> (x*y=w1019:dbl[][])
                n414 = To Unsigned Byte Integer "Normalised to 8 bit data"(number=w1019) -> (unsigned 8bit integer=w1017:u8[][])
              }
              frame Enabled {
                n415 = Array Max & Min(array=w1028) -> (min value=w1030:i32)  [unwired: 3 out]
                n416 = Negate(x=w1030) -> (-x=w1029:i32)
                n417 = Add(x=w1028, y=w1029) -> (x+y=w1027:i32[][])
                n418 = Absolute Value(x=w1033) -> (abs(x)=w1026:i32)
                n419 = Divide(x=w1027, y=w1026) -> (x/y=w1035:dbl[][])
                n420 = Multiply(x=w1035, y=65535.0 ("Numeric")) -> (x*y=w1032:dbl[][])
                n421 = To Unsigned Word Integer(number=w1032) -> (unsigned 16bit integer=w1031:u16[][])
              }
            }
            n422 = property class="ImageControl"(reference=w1008, "16-bit Display Conversion Method"=w1013, "16-bit Display Maximum Value"=w1015) -> (reference out=w1012:refnum<vi>, error out=w1011:errorcluster)  [unwired: 1 in]
            n423 = property class="ImageControl"(reference=w1012, error in=w1011, "16-bit Display Minimum Value"=w1005) -> (reference out=w1009:refnum<vi>, error out=w1010:errorcluster)
            n424 = Close Reference(reference=w1009, error in (no error)=w1010) -> ()  [unwired: 1 out]
            n425 = call "IMAQ ArrayToImage"("Image Pixels (U16)"=w996, "Image"=w1003) -> ("Image Out"=w1000:T6)  [unwired: 8 in, 1 out]
            n426 = call "IMAQ Copy"("Image Dst"=w1002, "Image Src"=w1000) -> ("Image Dst Out"=w1001:T6)  [unwired: 4 in, 1 out]
          }
        }
      }
      event "Imaging Path Histogram": Value Change {
        w1073 = u32 14 items=["Default"=10, "Most Significant Bits"=11, "Full Dynamic"=12, "Downshift"=13, "Given Range"=14, "90% Dynamic"=15, "Given Percent Range"=16] ("16-bit Display Mapping:Conversion Method")
        n427 = event-data() -> ("NewVal"=w1090:T8)  [unwired: 1 in]
        n428 = property class="Bool (strict)"(reference=w1079) -> (reference out=w1082:refnum<vi>, error out=w1081:errorcluster, "Value"=w1080:T11)  [unwired: 1 in]
        n429 = control-ref of="Imaging Path Image"() -> (w1087:refnum<vi>)
        n430 = control-ref of="Min Max (Blue)"() -> (w1086:refnum<vi>)
        n431 = Unbundle By Name(w1090) -> ("auto scale\n      Blue"=w1088:bool)
        n432 = control-ref of="Histogram"() -> (w1066:refnum<vi>)
        n433 = property class="Bool (strict)"(reference=w1082, error in=w1081, "Val(Sgnl)"=w1080) -> ()  [unwired: 2 out]
        n434 = call "IMAQ ImageToArray"("Image"=w1067) -> ("Image Pixels (I16)"=w1061:i16[][])  [unwired: 3 in, 4 out]
        n435 = call "IMAQ Histograph"("Image"=w1067) -> ("Histogram Graph"=w1065:T22)  [unwired: 7 in, 3 out]
        n436 = case shown="False" w1088 {
          tunnel: w1061 -> [w1120 w1141]
          tunnel: [w1121 w1131] -> w1076
          tunnel: [w1122 w1132] -> w1075
          tunnel: w1086 -> [w1128 w1136]
          tunnel: [w1120 w1141] -> w1062
          tunnel: w1066 -> [w1123 w1138]
          tunnel: w1065 -> [w1124 w1137]
          frame False {
            n437 = property class="Slide (strict)"(reference=w1128) -> (reference out=w1127:refnum<vi>, error out=w1130:errorcluster, "Value"=w1129:cluster{i16, i16})  [unwired: 1 in]
            n438 = Close Reference(reference=w1127, error in (no error)=w1130) -> ()  [unwired: 1 out]
            n439 = Unbundle(w1129) -> (w1122:i16, w1121:i16)
            n440 = property class="WFGraph (strict)"(reference=w1123, "Value"=w1124, "XScale.Minimum"=w1122, "XScale.Maximum"=w1121) -> (reference out=w1126:refnum<vi>, error out=w1125:errorcluster)  [unwired: 1 in]
            n441 = Close Reference(reference=w1126, error in (no error)=w1125) -> ()  [unwired: 1 out]
          }
          frame True {
            n442 = Array Max & Min(array=w1141) -> (max value=w1131:i16, min value=w1132:i16)  [unwired: 2 out]
            n443 = Bundle(w1132, w1131) -> (w1134:cluster{i16, i16})  [unwired: 1 in]
            n444 = property class="WFGraph (strict)"(reference=w1138, "Value"=w1137, "XScale.Minimum"=w1132, "XScale.Maximum"=w1131) -> (reference out=w1140:refnum<vi>, error out=w1139:errorcluster)  [unwired: 1 in]
            n445 = property class="Slide (strict)"(reference=w1136, "Value"=w1134, "Scale.Minimum"=w1132, "Scale.Maximum"=w1131) -> (reference out=w1135:refnum<vi>, error out=w1133:errorcluster)  [unwired: 1 in]
            n446 = Close Reference(reference=w1135, error in (no error)=w1133) -> ()  [unwired: 1 out]
            n447 = Close Reference(reference=w1140, error in (no error)=w1139) -> ()  [unwired: 1 out]
          }
        }
        n448 = To Long Integer(number=w1075) -> (32bit integer=w1059:i32)
        n449 = To Long Integer(number=w1076) -> (32bit integer=w1060:i32)
        n450 = To Long Integer(number=w1062) -> (32bit integer=w1058:i32[][])
        n451 = property class="ImageControl"(reference=w1087, "16-bit Display Conversion Method"=w1073, "16-bit Display Maximum Value"=w1076) -> (reference out=w1072:refnum<vi>, error out=w1071:errorcluster)  [unwired: 1 in]
        n452 = Subtract "Data range"(x=w1060, y=w1059) -> (x-y=w1074:i32)
        n453 = disable-structure shown="Enabled" {
          disable-tunnel: w1067 -> [w1116 w1119]
          disable-tunnel: [w1115 w1119] -> w1068
          frame Disabled {
            n454 = call "overlay_grid.vi"("no of grid lines"=1, "Color (red)"=u32 6618880 ("Color"), "Image In"=w1116) -> ("Image Out"=w1115:T6)  [unwired: 2 in]
          }
          frame Enabled {
            # "no cross-hair required.\nFP grid function can be used."
          }
        }
        n455 = disable-structure shown="Enabled" {
          disable-tunnel: [w1103 w1111] -> w1064
          disable-tunnel: w1074 -> [w1099 w1107]
          disable-tunnel: w1058 -> [_ w1105]
          frame Disabled {
            # "Make values positive; start from 0"
            # "compress data (lossy)"
            n456 = Array Max & Min() -> (array=w1100:dbl[], min value=w1102:dbl)  [unwired: 3 out]
            n457 = Negate(x=w1102) -> (-x=w1101:dbl)
            n458 = Add(x=w1100, y=w1101) -> (x+y=w1104:dbl)
            n459 = Divide(x=w1104, y=w1099) -> (x/y=w1098:dbl)
            n460 = Multiply(x=w1098, y=255.0 ("Numeric")) -> (x*y=w1096:dbl)
            n461 = To Unsigned Byte Integer "Normalised to 8 bit data"(number=w1096) -> (unsigned 8bit integer=w1103:u8)
          }
          frame Enabled {
            n462 = Array Max & Min(array=w1105) -> (min value=w1110:i32)  [unwired: 3 out]
            n463 = Negate(x=w1110) -> (-x=w1109:i32)
            n464 = Add(x=w1105, y=w1109) -> (x+y=w1108:i32[][])
            n465 = Absolute Value(x=w1107) -> (abs(x)=w1106:i32)
            n466 = Divide(x=w1108, y=w1106) -> (x/y=w1114:dbl[][])
            n467 = Multiply(x=w1114, y=65535.0 ("Numeric")) -> (x*y=w1112:dbl[][])
            n468 = To Unsigned Word Integer(number=w1112) -> (unsigned 16bit integer=w1111:u16[][])
          }
        }
        n469 = property class="ImageControl"(reference=w1072, error in=w1071, "16-bit Display Minimum Value"=w1075) -> (reference out=w1069:refnum<vi>, error out=w1070:errorcluster)
        n470 = Close Reference(reference=w1069, error in (no error)=w1070) -> ()  [unwired: 1 out]
        n471 = call "IMAQ ArrayToImage"("Image Pixels (U16)"=w1064, "Image"=w1077) -> ("Image Out"=w1084:T6)  [unwired: 8 in, 1 out]
      }
      event "Linear Zoom", "X-Offset (Pixels)", "Non Linear Stretch", "Sinusoidal Phase Correction\n(radians)", "Y-Offset (Pixels)": Value Change {
        # "Valid Image?"
        n472 = event-data() -> ()  [unwired: 1 in, 1 out]
        n473 = call "IMAQ Copy"("Image Dst"=w1154, "Image Src"=w1156) -> ("Image Dst Out"=w1157:T6)  [unwired: 4 in, 1 out]
        n474 = call "IMAQ GetImageSize"("Image"=w1156) -> ("Y Resolution"=w1155:i32)  [unwired: 3 in, 2 out]
        n475 = case shown="Default" w1155 {
          tunnel: [w1163 w1183] -> w1150
          tunnel: w1157 -> [_ w1193]
          tunnel: w1154 -> [w1163 _]
          tunnel: [_ w1178] -> w1147
          tunnel: [_ w1184] -> w1148
          tunnel: w1146 -> [_ _]
          tunnel: w1145 -> [_ w1170]
          tunnel: w1143 -> [_ w1175]
          tunnel: w1142 -> [_ w1192]
          frame 0 {
          }
          frame Default {
            w1191 = 0 ("index")
            # "Starting Pixel distribution (Linear)"
            n476 = call "IMAQ GetImageSize"("Image"=w1193) -> ("Y Resolution"=w1190:i32, "X Resolution"=w1177:i32)  [unwired: 3 in, 1 out]
            n477 = property on="Linear Zoom" class="Clust (strict)"() -> ("Value"=w1185:cluster{"X.Zoom":dbl, "Y.Zoom":dbl})  [unwired: 2 in, 2 out]
            n478 = Array Subset(array=w1192, index=w1191, length=w1177) -> (w1182:i16[])
            n479 = Array Subset(array=w1192, index=w1191, length=w1190) -> (w1189:i16[])
            n480 = property on="X-Offset (Pixels)" class="Slide (strict)"() -> ("Value"=w1196:i32)  [unwired: 2 in, 2 out]
            n481 = property on="Y-Offset (Pixels)" class="Slide (strict)"() -> ("Value"=w1197:i32)  [unwired: 2 in, 2 out]
            n482 = Unbundle By Name(w1185) -> ("X.Zoom"=w1179:dbl, "Y.Zoom"=w1171:dbl)
            n483 = disable-structure shown="Enabled" {
              disable-tunnel: [w1231 w1249] -> w1201
              disable-tunnel: [w1230 w1248] -> w1200
              disable-tunnel: [w1229 w1246] -> w1199
              disable-tunnel: [w1228 w1245] -> w1198
              disable-tunnel: w1197 -> [w1227 w1245]
              disable-tunnel: w1196 -> [w1226 w1246]
              disable-tunnel: [w1225 w1247] -> w1194
              disable-tunnel: w1193 -> [w1224 w1247]
              disable-tunnel: w1189 -> [w1223 w1248]
              disable-tunnel: w1182 -> [w1222 w1249]
              disable-tunnel: "Flip" -> [w1221 _]
              frame Disabled {
                n484 = case shown="False" w1221 {
                  tunnel: w1224 -> [w1236 w1243]
                  tunnel: [w1236 w1242] -> w1225
                  tunnel: w1223 -> [w1232 w1240]
                  tunnel: w1222 -> [w1233 w1241]
                  tunnel: [w1232 w1240] -> w1230
                  tunnel: w1226 -> [w1235 w1239]
                  tunnel: w1227 -> [w1234 w1238]
                  tunnel: [w1235 w1239] -> w1229
                  tunnel: [w1234 w1238] -> w1228
                  tunnel: [w1233 w1237] -> w1231
                  frame False {
                  }
                  frame True {
                    w1244 = u32 1 items=["Horizontal", "Vertical", "Central", "1st Diagonal", "2nd Diagonal"] ("Type of Symmetry")
                    n485 = Reverse 1D Array(array=w1241) -> (reversed array=w1237:i16[])
                    n486 = call "IMAQ Symmetry"("Type of Symmetry"=w1244, "Image Src"=w1243) -> ("Image Dst Out"=w1242:T6)  [unwired: 3 in, 1 out]
                  }
                }
              }
              frame Enabled {
                # "FLIP Disabled!"
              }
            }
            n487 = disable-structure shown="Enabled" {
              disable-tunnel: w1199 -> [w1213 w1220]
              disable-tunnel: [w1212 w1220] -> w1195
              disable-tunnel: w1170 -> [w1211 _]
              frame Disabled {
                n488 = case shown="\"ImagingGalvoCalibration\"" w1211 {
                  tunnel: w1213 -> [w1214 w1216]
                  tunnel: [w1214 w1215] -> w1212
                  frame "ImagingResoCalibration", Default {
                  }
                  frame "ImagingGalvoCalibration" {
                    n489 = disable-structure shown="Enabled" {
                      disable-tunnel: w1216 -> [w1218 w1219]
                      disable-tunnel: [w1217 w1219] -> w1215
                      frame Enabled {
                        n490 = Negate(x=w1218) -> (-x=w1217:i32)
                      }
                      frame Disabled {
                      }
                    }
                  }
                }
              }
              frame Enabled {
                # "Offset inversion disabled!\n\nThis is required if an image flip is carried out in software"
              }
            }
            n491 = call "IMAQ Shift"("Color Replace Value"=u32 16711680, "YOffset"=w1198, "Replace Value"=sgl 100.0, "XOffset"=w1199, "Image Src"=w1194) -> ("Image Dst Out"=w1172:T6)  [unwired: 5 in, 1 out]
            n492 = property on="Sinusoidal Phase Correction\n(radians)" class="Slide (strict)"() -> ("Value"=w1176:dbl)  [unwired: 2 in, 2 out]
            n493 = To Word Integer(number=w1198) -> (16bit integer=w1164:i16)
            n494 = Subtract(x=w1200, y=w1164) -> (x-y=w1173:i16[])
            n495 = To Word Integer(number=w1195) -> (16bit integer=w1165:i16)
            n496 = Subtract(x=w1201, y=w1165) -> (x-y=w1174:i16[])
            n497 = call "Test__Zoom Corection.vi"("Reference Image IN"=w1172, "Modified Image IN"=w1172, "Flipped?"="Flip", "X-Stretch"=w1179, "Y-Stretch"=w1171, "X Indices IN"=w1174, "Y Indices IN"=w1173) -> ("Modified Image OUT"=w1166:T6, "X Indices OUT"=w1168:i16[], "Y Indices OUT"=w1178:i16[], "X_Pixels Dropped (if ZOOM <1)"=w1167:T25)  [unwired: 5 in]
            n498 = case shown="\"ImagingResoCalibration\"" w1170 {
              tunnel: w1168 -> [w1203 w1210]
              tunnel: w1167 -> [_ w1209]
              tunnel: w1166 -> [w1202 w1208]
              tunnel: w1175 -> [_ w1207]
              tunnel: w1176 -> [_ w1206]
              tunnel: [w1203 w1205] -> w1184
              tunnel: [w1202 w1204] -> w1183
              frame Default {
              }
              frame "ImagingResoCalibration" {
                n499 = call "Resonant X-Stretch Compensation.vi"("Excess X_Pixels (if ZOOM <1)"=w1209, "Reso Phase correction factor"=w1206, "Start Delay (Ticks)"=w1207, "X Pixel Array IN"=w1210, "Image Ref IN"=w1208) -> ("X-Stretched Array OUT"=w1205:i16[], "Corrected Image Out"=w1204:T6)  [unwired: 5 in]
              }
            }
            n500 = Bundle(w1182, "X-Stretched Array OUT"=w1184) -> (w1187:cluster{i16[], "X-Stretched Array OUT":i16[]})  [unwired: 1 in]
            n501 = Bundle(w1189, "Y Indices OUT"=w1178) -> (w1188:cluster{i16[], "Y Indices OUT":i16[]})  [unwired: 1 in]
            n502 = Build Array(w1187, w1188) -> (→"Relationship between initial pixels and pixels after transformation":cluster{i16[], "Y Indices OUT":i16[]}[])
          }
        }
        n503 = local write "X-Pixel Mapping"(w1148) -> ()
        n504 = local write "Y-Pixel Mapping"(w1147) -> ()
        n505 = call "Red-Blue Overlay with Select.vi"("RGB IMageRefnum IN"=w1151, "Blue Channel Refnum"=w1149, "Enable Blue?"="Blue", "Red Channel Refnum"=w1150, "Enable Red?"="Red") -> ("RGB Image Refnum out OUT"=w1144:T6)  [unwired: 6 in]
        "Red-Blue Overlay" <- w1144
      }
      event "Red", "Blue": Value Change {
        # "Trigger an event"
        n506 = event-data() -> ()  [unwired: 1 in, 1 out]
        n507 = property class="Bool (strict)"(reference=w1252) -> (reference out=w1255:refnum<vi>, error out=w1254:errorcluster, "Value"=w1253:T11)  [unwired: 1 in]
        n508 = property class="Bool (strict)"(reference=w1255, error in=w1254, "Val(Sgnl)"=w1253) -> ()  [unwired: 2 out]
      }
      event Value Change {
        n509 = event-data() -> ()  [unwired: 1 in, 1 out]
        n510 = call "Dialog_Clear Calibration.vi"() -> ("Clear Type Requested (Galvo; Reso; Both; None)"=w1270:string)  [unwired: 11 in]
        n511 = case "Select files to write" shown="\"Both\"" w1270 {
          tunnel: w1269 -> [_ w1314 w1321 w1332]
          tunnel: [path[] [] w1311 w1320 w1332] -> w1268
          tunnel: w1267 -> [w1304 w1308 w1316 w1329]
          tunnel: [w1304 w1306 w1315 w1324] -> w1266
          frame "None", Default {
          }
          frame "Galvo" {
            n512 = Index Array(array=w1314, index=0) -> (element=w1312:path)
            n513 = Replace Array Subset(array=w1308, new element="", index (row)=1, index (col)=1 ("disabled index (col)")) -> (w1306:string[][])
            n514 = Build Array(w1312) -> (w1311:path[])
          }
          frame "Reso" {
            n515 = Index Array(array=w1321, index=1) -> (element=w1322:path)
            n516 = Replace Array Subset(array=w1316, new element="", index (row)=2, index (col)=1 ("disabled index (col)")) -> (w1315:string[][])
            n517 = Build Array(w1322) -> (w1320:path[])
          }
          frame "Both" {
            w1325 = ""
            n518 = Replace Array Subset(array=w1329, new element=w1325, index (row)=1, index (col)=1 ("disabled index (col)")) -> (w1326:string[][])
            n519 = Replace Array Subset(array=w1326, new element=w1325, index (row)=2, index (col)=1 ("disabled index (col)")) -> (w1324:string[][])
          }
        }
        n520 = for "Iterate through all files to be written" {
          tunnel: w1268 -> [w1288] mode=indexing
          n521 = call <vilib>:"Open Config Data.vi"("configuration file path"=w1288) -> ("error out"=w1286:errorcluster, "refnum"=w1287:T23)  [unwired: 8 in, 1 out]
          n522 = call <vilib>:"Get Section Names.vi"("error in (no error)"=w1286, "refnum"=w1287) -> ("error out"=w1284:errorcluster, "section names"=w1285:string[], "refnum out"=w1282:T23)  [unwired: 7 in]
          n523 = for "Iterate through all section" {
            tunnel: w1285 -> [w1293] mode=indexing
            tunnel: w1282 -> [w1295]
            tunnel: w1284 -> [w1294]
            tunnel: [w1289] -> w1283
            w1290 = "SystemType"  # Don't delete system type!
            n524 = call <vilib>:"Get Key Names.vi"("section"=w1293, "error in (no error)"=w1294, "refnum"=w1295) -> ("error out"=w1289:errorcluster, "key names"=w1291:string[], "refnum out"=w1292:T23)  [unwired: 5 in, 1 out]
            n525 = for "Iterate through Sections and delete" {
              tunnel: w1293 -> [w1300]
              tunnel: w1292 -> [w1299]
              tunnel: w1291 -> [w1297] mode=indexing
              tunnel: w1290 -> [w1298]
              n526 = Not Equal?(x=w1297, y=w1298) -> (x != y?=w1296:bool)
              n527 = case shown="True" w1296 {
                tunnel: w1300 -> [_ w1303]
                tunnel: w1299 -> [_ w1302]
                tunnel: w1297 -> [_ w1301]
                frame False {
                }
                frame True {
                  n528 = call <vilib>:"Remove Key.vi"("section"=w1303, "key"=w1301, "refnum"=w1302) -> ()  [unwired: 6 in, 3 out]
                }
              }
            }
          }
          n529 = call <vilib>:"Close Config Data.vi"("error in (no error)"=w1283, "refnum"=w1282) -> ()  [unwired: 8 in, 2 out]
        }
      }
    }
    "Reference Image (From Uncaging Path)" <- w90
    "Imaging Path Image" <- w89
  }
  n530 = flat-sequence {
    tunnel: w18 -> [_]
    frame #0 {
      n531 = control-ref of="This VI"() -> (w1333:refnum<vi>)
      n532 = invoke class="VI" method="FP.Close"(reference=w1333) -> ()  [unwired: 2 in, 3 out]
    }
  }
